vi "日志信息出发送队列 (子VI).vi"() -> (0 "错误输出":errorcluster)   [LabVIEW 2016, in "数据传输系统-03.lvlib"]
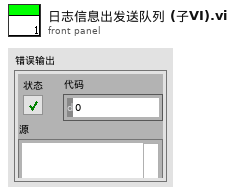
[diagram p1: front panel]
types:
  T1 = enum16{"空白测试", "跨度核查", "标样核查", "加标回收", "平行样", "集成干预"}
  T2 = cluster{"氨氮零点核查索引起始时间":string, "总磷零点核查索引起始时间":string, "总氮零点核查索引起始时间":string, "CODMn零点核查索引起始时间":string, "CODCr零点核查索引起始时间":string, "亚硝酸盐零点核查索引起始时间":string, "硫化物零点核查索引起始时间":string, "ORP零点核查索引起始时间":string, "氟化物零点核查索引起始时间":string}
  T3 = cluster{"数组[0]":string, "数组[1]":string, "数组[2]":string, "数组[3]":string, "数组[4]":string, "数组[5]":string, "数组[6]":string, "数组[7]":string, "数组[8]":string}
  T4 = cluster{"PH":string[][], "CODCr":string[][], "氨氮":string[][], "CODMn":string[][], "总氮":string[][], "总磷":string[][], "电导率":string[][], "水温":string[][], "DO":string[][], "浊度":string[][], "叶绿素":string[][], "藻密度":string[][], "铜":string[][], "盐度":string[][], "水位":string[][], "流速":string[][], "瞬时流量":string[][], "累积流量":string[][], "亚硝酸盐":string[][], "硫化物":string[][], "ORP":string[][], "铅":string[][], "镉":string[][], "锌":string[][], "镍":string[][], "锰":string[][], "汞":string[][], "气温":string[][], "气压":string[][], "风速":string[][], "风向":string[][], "盐度 2":string[][], "磷酸盐":string[][], "硝氮":string[][], "氟化物":string[][]}
  T5 = cluster{"氨氮跨度核查索引起始时间":string, "总磷跨度核查索引起始时间":string, "总氮跨度核查索引起始时间":string, "CODMn跨度核查索引起始时间":string, "CODCr跨度核查索引起始时间":string, "亚硝酸盐跨度核查索引起始时间":string, "硫化物跨度核查索引起始时间":string, "ORP跨度核查索引起始时间":string, "氟化物跨度核查索引起始时间":string}
  T6 = cluster{"氨氮标样核查索引起始时间":string, "总磷标样核查索引起始时间":string, "总氮标样核查索引起始时间":string, "CODMn标样核查索引起始时间":string, "CODCr标样核查索引起始时间":string, "DO标样核查索引起始时间":string, "PH标样核查索引起始时间":string, "比电导率标样核查索引起始时间":string, "水温标样核查索引起始时间":string, "浊度标样核查索引起始时间":string, "叶绿素a标样核查索引起始时间":string, "藻密度标样核查索引起始时间":string, "亚硝酸盐标样核查索引起始时间":string, "硫化物标样核查索引起始时间":string, "ORP标样核查索引起始时间":string, "氟化物标样核查索引起始时间":string}
  T7 = cluster{"数组[0]":string, "数组[1]":string, "数组[2]":string, "数组[3]":string, "数组[4]":string, "数组[5]":string, "数组[6]":string, "数组[7]":string, "数组[8]":string, "数组[9]":string, "数组[10]":string, "数组[11]":string, "数组[12]":string, "数组[13]":string, "数组[14]":string, "数组[15]":string}
  T8 = cluster{"氨氮加标回收索引起始时间":string, "总磷加标回收索引起始时间":string, "总氮加标回收索引起始时间":string, "CODMn加标回收索引起始时间":string, "CODCr加标回收索引起始时间":string, "氟化物加标回收索引起始时间":string}
  T9 = cluster{"[0]":string, "[1]":string, "[2]":string, "[3]":string, "[4]":string, "[5]":string}
  T10 = cluster{"氨氮平行样索引起始时间":string, "总磷平行样索引起始时间":string, "总氮平行样索引起始时间":string, "CODMn平行样索引起始时间":string, "CODCr平行样索引起始时间":string, "氟化物平行样索引起始时间":string}
  T11 = cluster{"氨氮集成干预索引起始时间":string, "总磷集成干预索引起始时间":string, "总氮集成干预索引起始时间":string, "CODMn集成干预索引起始时间":string, "CODCr集成干预索引起始时间":string, "DO集成干预索引起始时间":string, "PH集成干预索引起始时间":string, "比电导率集成干预索引起始时间":string, "水温集成干预索引起始时间":string, "浊度集成干预索引起始时间":string, "叶绿素a集成干预索引起始时间":string, "藻密度集成干预索引起始时间":string, "亚硝酸盐集成干预索引起始时间":string, "硫化物集成干预索引起始时间":string, "ORP集成干预索引起始时间":string, "氟化物集成干预索引起始时间":string}
  T12 = cluster{"[0]":string, "[1]":string, "[2]":string, "[3]":string, "[4]":string, "[5]":string, "[6]":string, "[7]":string, "[8]":string, "[9]":string, "[10]":string, "[11]":string, "[12]":string, "[13]":string, "[14]":string, "[15]":string}
  T13 = cluster{"氨氮仪器日志索引起始时间":string, "总磷仪器日志索引起始时间":string, "总氮仪器日志索引起始时间":string, "CODMn仪器日志索引起始时间":string, "CODCr仪器日志索引起始时间":string, "系统仪器日志索引起始时间":string, "氟化物仪器日志索引起始时间":string}
  T14 = cluster{"[0]":string, "[1]":string, "[2]":string, "[3]":string, "[4]":string, "[5]":string, "[6]":string}
  T15 = cluster{"氨氮报警信息索引起始时间":string, "总磷报警信息索引起始时间":string, "总氮报警信息索引起始时间":string, "CODMn报警信息索引起始时间":string, "CODCr报警信息索引起始时间":string, "DO报警信息索引起始时间":string, "PH报警信息索引起始时间":string, "比电导率报警信息索引起始时间":string, "水温报警信息索引起始时间":string, "浊度报警信息索引起始时间":string, "叶绿素报警信息索引起始时间":string, "系统报警信息索引起始时间":string, "氟化物报警信息索引起始时间":string}
  T16 = cluster{"[0]":string, "[1]":string, "[2]":string, "[3]":string, "[4]":string, "[5]":string, "[6]":string, "[7]":string, "[8]":string, "[9]":string, "[10]":string, "[11]":string, "[12]":string}
  T17 = cluster{"氨氮仪器参数索引起始时间":string, "总磷仪器参数索引起始时间":string, "总氮仪器参数索引起始时间":string, "CODMn仪器参数索引起始时间":string, "CODCr仪器参数索引起始时间":string, "DO仪器参数索引起始时间":string, "PH仪器参数索引起始时间":string, "比电导率仪器参数索引起始时间":string, "水温仪器参数索引起始时间":string, "浊度仪器参数索引起始时间":string, "叶绿素a仪器参数索引起始时间":string, "藻密度仪器参数索引起始时间":string, "ORP仪器参数索引起始时间":string, "氟化物仪器参数索引起始时间":string}
  T18 = cluster{"[0]":string, "[1]":string, "[2]":string, "[3]":string, "[4]":string, "[5]":string, "[6]":string, "[7]":string, "[8]":string, "[9]":string, "[10]":string, "[11]":string, "[12]":string, "[13]":string}
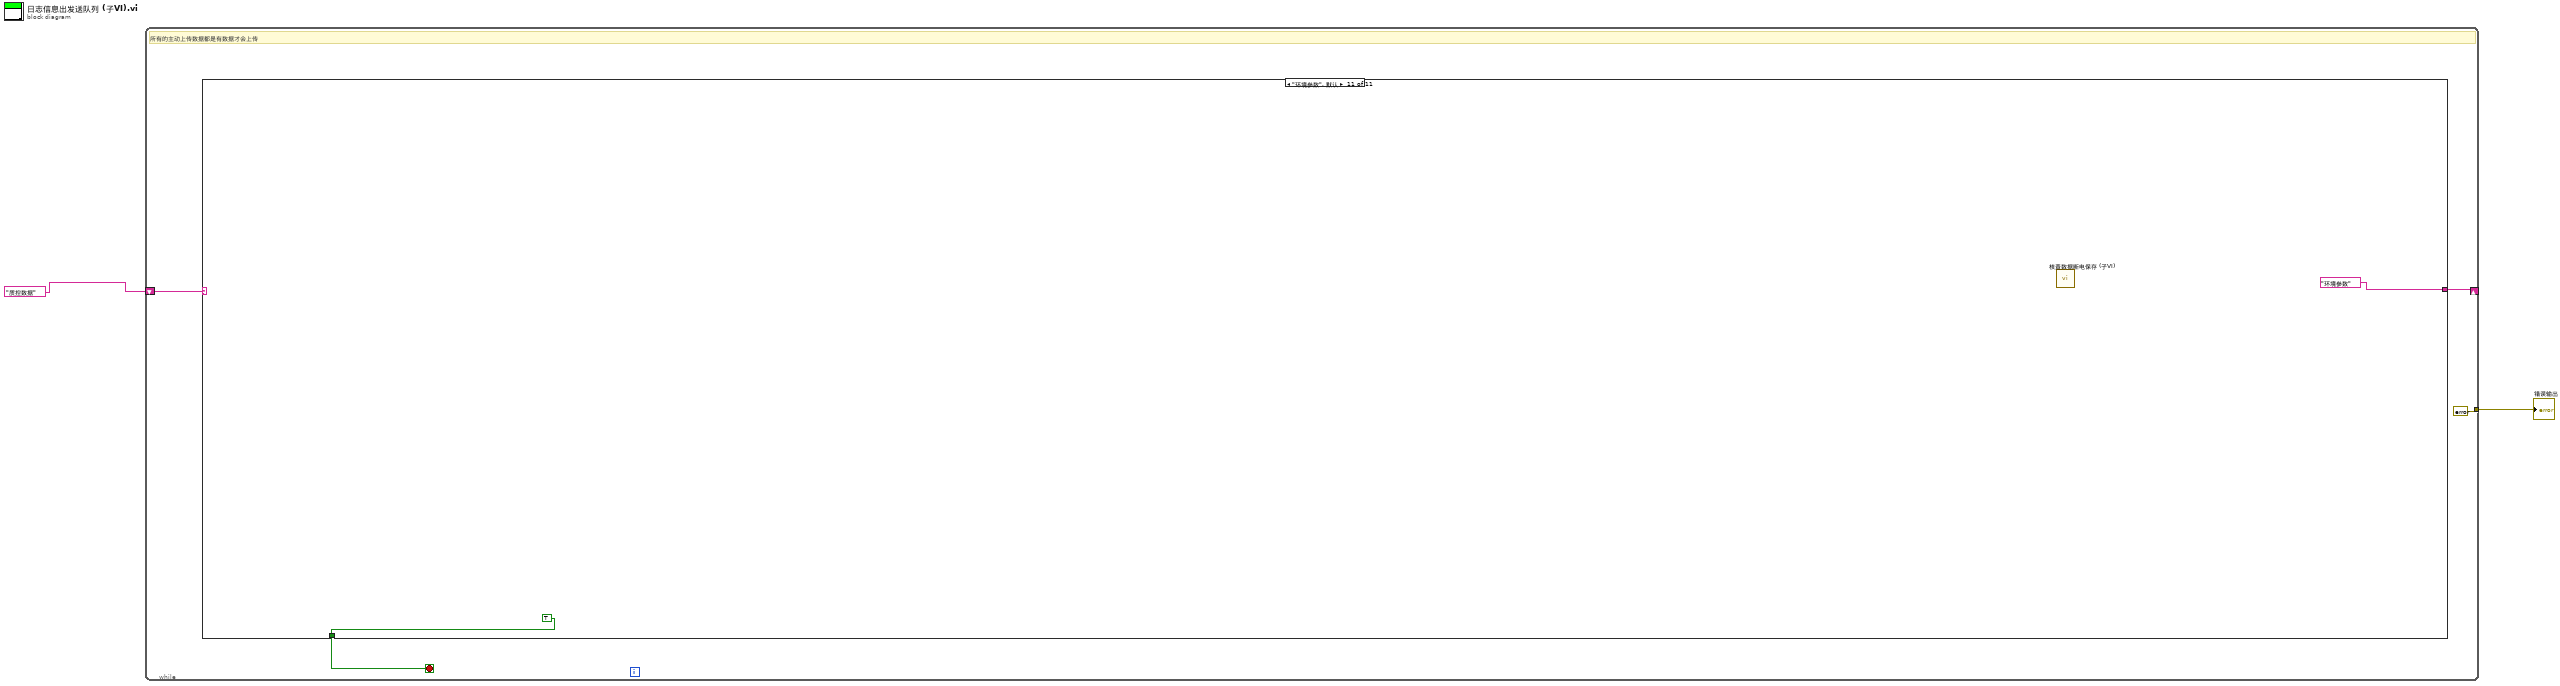
[diagram p0: block diagram]
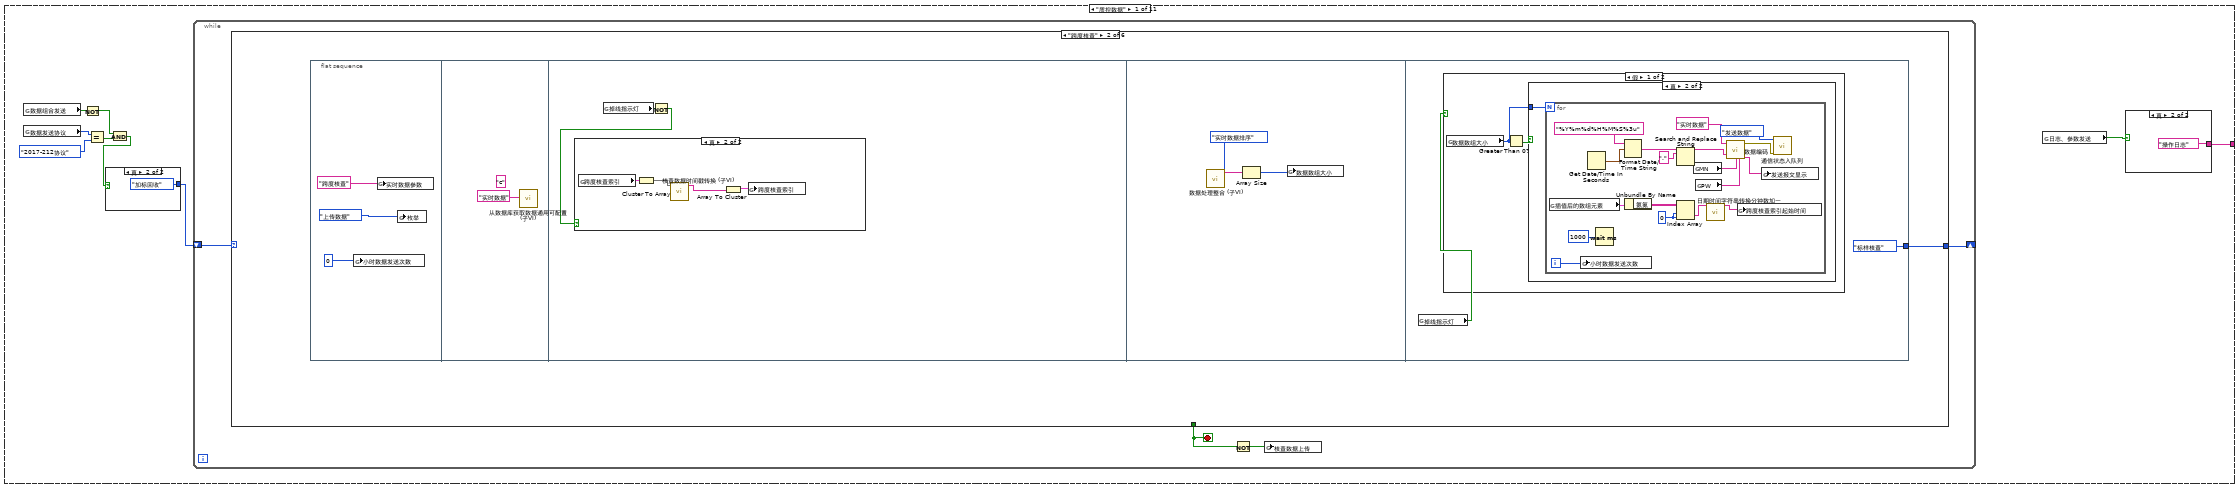
[diagram p2: hidden frame]
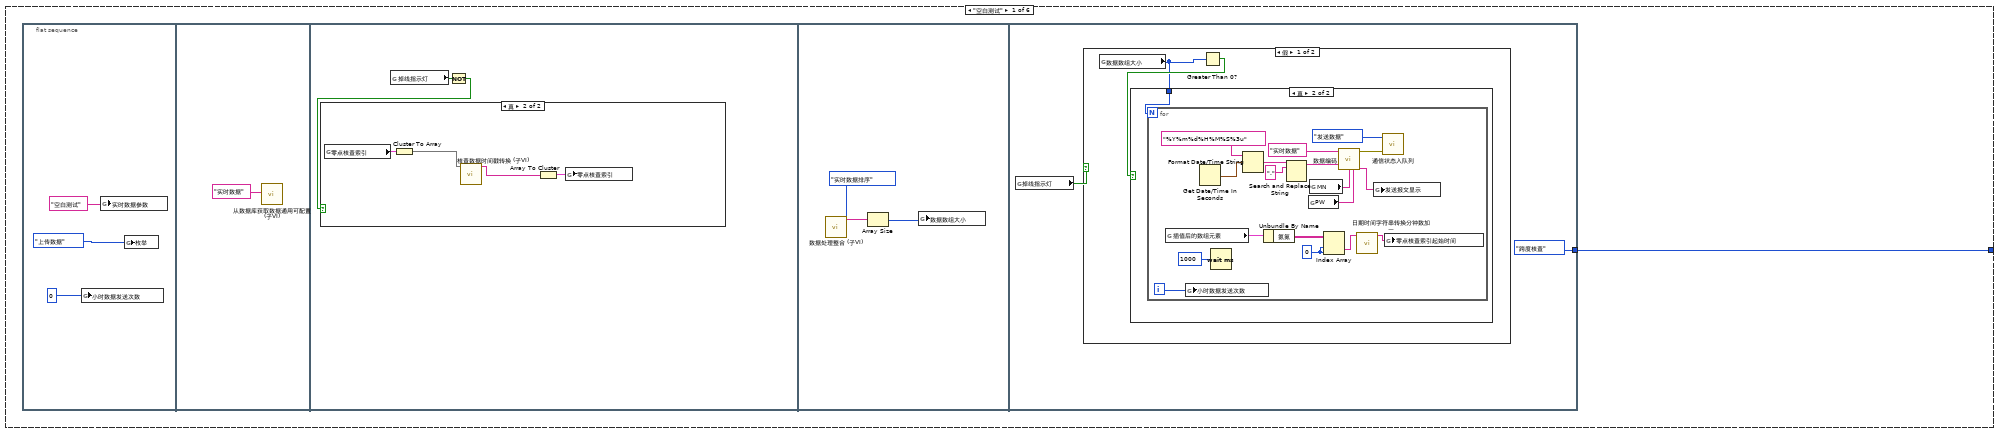
[diagram p3: hidden frame]
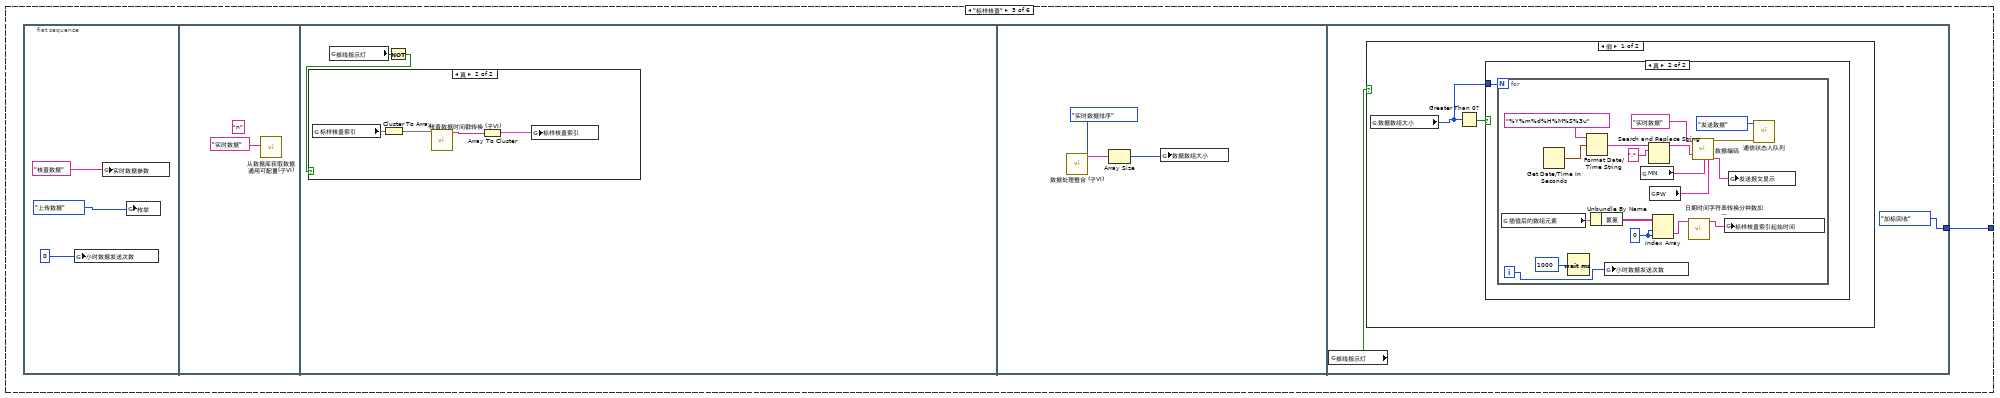
[diagram p10: hidden frame]
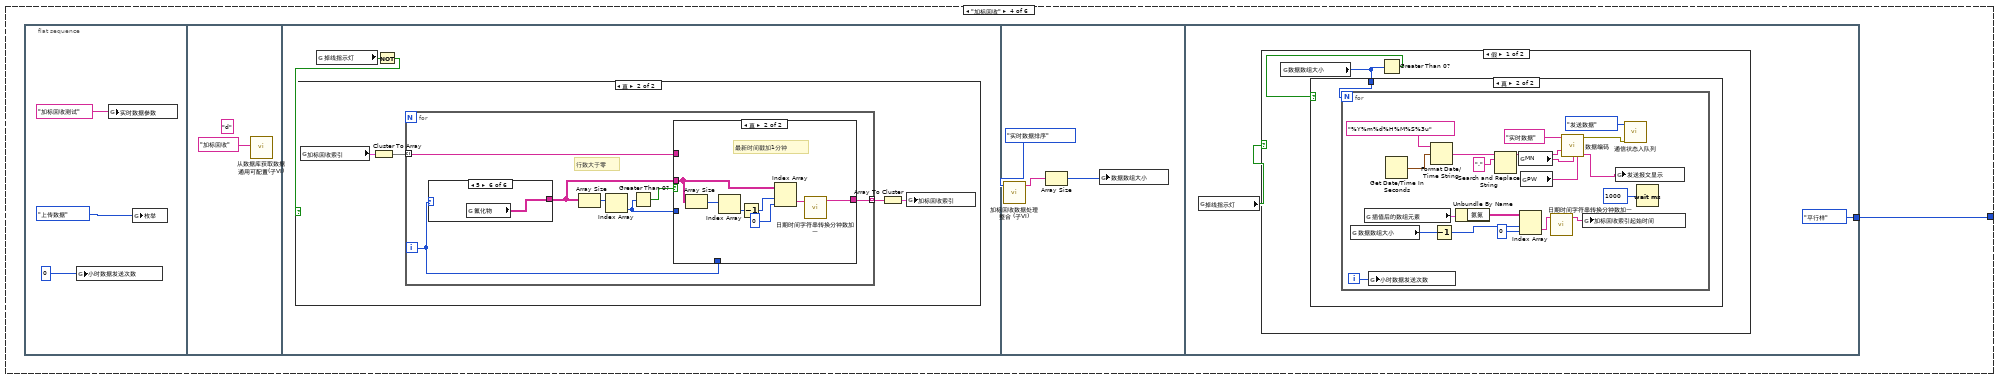
[diagram p14: hidden frame]
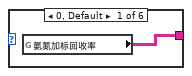
[diagram p16: hidden frame]
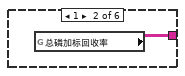
[diagram p17: hidden frame]
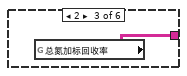
[diagram p18: hidden frame]
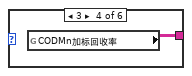
[diagram p19: hidden frame]
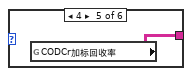
[diagram p20: hidden frame]
diagram:
  n1 = while "While循环" {
    shift-right: [w5] -> _
    shift-left: "质控数据" ("组合框") -> [w6]
    tunnel: [errorcluster {"status"=FALSE, "code"=0, "source"=""} ("错误输出")] -> w2
    stop <- w3 stop-if-true
    # "所有的主动上传数据都是有数据才会上传"
    n2 = case shown="\"环境参数\", 默认" w6 {
      tunnel: [w15 w312 "系统状态" ("组合框") w414 "测量周期" ("组合框") "超标留样" ("组合框") "报警信息" ("组合框") w508 w574 "环境参数" ("组合框") "环境参数" ("组合框")] -> w5
      tunnel: [_ _ _ _ _ _ _ _ _ _ TRUE] -> w3
      frame "质控数据" {
        n3 = global read "断电保存全局.vi" "数据组合发送"() -> (w10:bool)
        n4 = global read "断电保存全局.vi" "数据发送协议"() -> (w13:enum16{"2005-212协议", "2017-212协议"})
        n5 = Not(x=w10) -> (.not. x?=w9:bool)
        n6 = Equal?(x=w13, y=enum16{"2005-212协议", "2017-212协议"}."2017-212协议" ("数据发送协议")) -> (x = y?=w11:bool)
        n7 = And(x=w9, y=w11) -> (x .and. y?=w8:bool)
        n8 = case shown="真" w8 {
          tunnel: [T1."空白测试" T1."加标回收"] -> w7
          frame False {
          }
          frame True {
          }
        }
        n9 = while {
          shift-right: [w18] -> _
          shift-left: w7 -> [w19]
          stop <- w16 stop-if-true
          n10 = case shown="\"跨度核查\"" w19 {
            tunnel: [_ _ _ _ _ TRUE] -> w16
            tunnel: [w20 w57 w94 w131 w191 w244] -> w18
            frame "空白测试" {
              n11 = flat-sequence {
                tunnel: [T1."跨度核查"] -> w20
                frame #0 {
                  n12 = global write "全局 小时数据发送次数.vi" "小时数据发送次数"(0 ("小时数据发送次数")) -> ()
                  n13 = global write "全局 实时数据参数.vi" "实时数据参数"("空白测试") -> ()
                  n14 = global write "全局1.vi" "枚举"(enum16{"返回请求应答", "上传数据", "返回执行结果"}."上传数据" ("枚举")) -> ()
                }
                frame #1 {
                  n15 = call "从数据库获取数据通用可配置(子VI).vi"("table输入"="实时数据" ("新元素/子数组")) -> ()  [unwired: 9 in, 2 out]
                }
                frame #2 {
                  n16 = global read "全局 数据发送重叠.vi" "掉线指示灯"() -> (w26:bool)
                  n17 = Not(x=w26) -> (.not. x?=w25:bool)
                  n18 = case shown="真" w25 {
                    frame False {
                    }
                    frame True {
                      n19 = global read "全局 时间2.vi" "零点核查索引"() -> (w30:T2)
                      n20 = Cluster To Array(cluster=w30) -> (array=w28:string[])
                      n21 = call "核查数据时间戳转换 (子VI).vi"("核查索引"=w28) -> ("数组"=w27:string[])  [unwired: 10 in]
                      n22 = Array To Cluster(array=w27) -> (cluster=w29:T3)
                      n23 = global write "全局 时间2.vi" "零点核查索引"(w29) -> ()
                    }
                  }
                }
                frame #3 {
                  n24 = call "数据处理整合 (子VI).vi"("枚举"=enum16{"实时数据排序", "小时数据排序"}."实时数据排序") -> ("已排序的数组"=w33:string[])  [unwired: 10 in]
                  n25 = Array Size(array=w33) -> (size(s)=w32:i32)
                  n26 = global write "全局 数据数组大小.vi" "数据数组大小"(w32) -> ()
                }
                frame #4 {
                  n27 = global read "全局 数据发送重叠.vi" "掉线指示灯"() -> (w35:bool)
                  n28 = case shown="假" w35 {
                    frame False {
                      n29 = global read "全局 数据数组大小.vi" "数据数组大小"() -> (w36:i32)
                      n30 = Greater Than 0?(x=w36) -> (x > 0?=w37:bool)
                      n31 = case shown="真" w37 {
                        tunnel: w36 -> [_ w38]
                        frame False {
                        }
                        frame True {
                          n32 = for {
                            N: w38 -> [_]
                            i -> [w39]
                            w51 = 0 ("禁用的索引 (列)")
                            n33 = global read "插值后的新数组.vi" "插值后的数组元素"() -> (w55:T4)
                            n34 = global write "全局 小时数据发送次数.vi" "小时数据发送次数"(w39) -> ()
                            n35 = Get Date/Time In Seconds() -> (seconds since 1Jan1904=w43:timestamp)
                            n36 = Wait (ms)(milliseconds to wait=u32 1000 ("等待时间（毫秒）")) -> ()  [unwired: 1 out]
                            n37 = Format Date/Time String(time format string (%c)="%Y%m%d%H%M%S%3u" ("时间格式字符串(%c)"), seconds (now)=w43) -> (date/time string=w42:string)  [unwired: 1 in]
                            n38 = Unbundle By Name(w55) -> ("氨氮"=w54:string[][])
                            n39 = Search and Replace String(input string=w42, search string="." ("搜索字符串")) -> (result string=w40:string)  [unwired: 6 in, 3 out]
                            n40 = global read "断电保存全局.vi" "PW"() -> (w47:string)
                            n41 = global read "断电保存全局.vi" "MN"() -> (w48:string)
                            n42 = Index Array(array=w54, index (row)=w51, index (col)=w51) -> (element=w53:string)
                            n43 = call "数据编码.vi"("table输入"="实时数据" ("新元素/子数组"), "QN"=w40, "MN"=w48, "PW"=w47) -> ("错误常量"=w46:errorcluster, "通讯包字符串"=w50:string)  [unwired: 10 in]
                            n44 = call "日期时间字符串转换分钟数加一.vi"("data[0]"=w53) -> ("日期/时间字符串"=w52:string)  [unwired: 10 in]
                            n45 = global write "全局1.vi" "发送报文显示"(w50) -> ()
                            n46 = call "通信状态入队列.vi"("错误输入（无错误）"=w46, "枚举"=enum16{"打开连接", "发送数据", "读取数据", "数据处理", "关闭连接"}."发送数据") -> ()  [unwired: 9 in, 1 out]
                            n47 = global write "全局 时间2.vi" "零点核查索引起始时间"(w52) -> ()
                          }
                        }
                      }
                    }
                    frame True {
                    }
                  }
                }
              }
            }
            frame "跨度核查" {
              n48 = flat-sequence {
                tunnel: [T1."标样核查"] -> w57
                frame #0 {
                  n49 = global write "全局 小时数据发送次数.vi" "小时数据发送次数"(0 ("小时数据发送次数")) -> ()
                  n50 = global write "全局 实时数据参数.vi" "实时数据参数"("跨度核查") -> ()
                  n51 = global write "全局1.vi" "枚举"(enum16{"返回请求应答", "上传数据", "返回执行结果"}."上传数据" ("枚举")) -> ()
                }
                frame #1 {
                  (unwired) "c" ("列队名（唯一）")
                  n52 = call "从数据库获取数据通用可配置(子VI).vi"("table输入"="实时数据" ("新元素/子数组")) -> ()  [unwired: 9 in, 2 out]
                }
                frame #2 {
                  n53 = global read "全局 数据发送重叠.vi" "掉线指示灯"() -> (w63:bool)
                  n54 = Not(x=w63) -> (.not. x?=w62:bool)
                  n55 = case shown="真" w62 {
                    frame False {
                    }
                    frame True {
                      n56 = global read "全局 时间2.vi" "跨度核查索引"() -> (w67:T5)
                      n57 = Cluster To Array(cluster=w67) -> (array=w65:string[])
                      n58 = call "核查数据时间戳转换 (子VI).vi"("核查索引"=w65) -> ("数组"=w64:string[])  [unwired: 10 in]
                      n59 = Array To Cluster(array=w64) -> (cluster=w66:T3)
                      n60 = global write "全局 时间2.vi" "跨度核查索引"(w66) -> ()
                    }
                  }
                }
                frame #3 {
                  n61 = call "数据处理整合 (子VI).vi"("枚举"=enum16{"实时数据排序", "小时数据排序"}."实时数据排序") -> ("已排序的数组"=w70:string[])  [unwired: 10 in]
                  n62 = Array Size(array=w70) -> (size(s)=w69:i32)
                  n63 = global write "全局 数据数组大小.vi" "数据数组大小"(w69) -> ()
                }
                frame #4 {
                  n64 = global read "全局 数据发送重叠.vi" "掉线指示灯"() -> (w72:bool)
                  n65 = case shown="假" w72 {
                    frame False {
                      n66 = global read "全局 数据数组大小.vi" "数据数组大小"() -> (w73:i32)
                      n67 = Greater Than 0?(x=w73) -> (x > 0?=w74:bool)
                      n68 = case shown="真" w74 {
                        tunnel: w73 -> [_ w75]
                        frame False {
                        }
                        frame True {
                          n69 = for {
                            N: w75 -> [_]
                            i -> [w76]
                            w88 = 0 ("禁用的索引 (列)")
                            n70 = global read "插值后的新数组.vi" "插值后的数组元素"() -> (w92:T4)
                            n71 = global write "全局 小时数据发送次数.vi" "小时数据发送次数"(w76) -> ()
                            n72 = Get Date/Time In Seconds() -> (seconds since 1Jan1904=w80:timestamp)
                            n73 = Wait (ms)(milliseconds to wait=u32 1000 ("等待时间（毫秒）")) -> ()  [unwired: 1 out]
                            n74 = Format Date/Time String(time format string (%c)="%Y%m%d%H%M%S%3u" ("时间格式字符串(%c)"), seconds (now)=w80) -> (date/time string=w79:string)  [unwired: 1 in]
                            n75 = Unbundle By Name(w92) -> ("氨氮"=w91:string[][])
                            n76 = Index Array(array=w91, index (row)=w88, index (col)=w88) -> (element=w90:string)
                            n77 = Search and Replace String(input string=w79, search string="." ("搜索字符串")) -> (result string=w77:string)  [unwired: 6 in, 3 out]
                            n78 = global read "断电保存全局.vi" "MN"() -> (w86:string)
                            n79 = global read "断电保存全局.vi" "PW"() -> (w85:string)
                            n80 = call "日期时间字符串转换分钟数加一.vi"("data[0]"=w90) -> ("日期/时间字符串"=w89:string)  [unwired: 10 in]
                            n81 = call "数据编码.vi"("table输入"="实时数据" ("新元素/子数组"), "QN"=w77, "MN"=w86, "PW"=w85) -> ("错误常量"=w83:errorcluster, "通讯包字符串"=w84:string)  [unwired: 10 in]
                            n82 = global write "全局 时间2.vi" "跨度核查索引起始时间"(w89) -> ()
                            n83 = global write "全局1.vi" "发送报文显示"(w84) -> ()
                            n84 = call "通信状态入队列.vi"("错误输入（无错误）"=w83, "枚举"=enum16{"打开连接", "发送数据", "读取数据", "数据处理", "关闭连接"}."发送数据") -> ()  [unwired: 9 in, 1 out]
                          }
                        }
                      }
                    }
                    frame True {
                    }
                  }
                }
              }
            }
            frame "标样核查" {
              n85 = flat-sequence {
                tunnel: [T1."加标回收"] -> w94
                frame #0 {
                  n86 = global write "全局 小时数据发送次数.vi" "小时数据发送次数"(0 ("小时数据发送次数")) -> ()
                  n87 = global write "全局 实时数据参数.vi" "实时数据参数"("核查数据") -> ()
                  n88 = global write "全局1.vi" "枚举"(enum16{"返回请求应答", "上传数据", "返回执行结果"}."上传数据" ("枚举")) -> ()
                }
                frame #1 {
                  (unwired) "n" ("列队名（唯一）")
                  n89 = call "从数据库获取数据通用可配置(子VI).vi"("table输入"="实时数据" ("新元素/子数组")) -> ()  [unwired: 9 in, 2 out]
                }
                frame #2 {
                  n90 = global read "全局 数据发送重叠.vi" "掉线指示灯"() -> (w100:bool)
                  n91 = Not(x=w100) -> (.not. x?=w99:bool)
                  n92 = case shown="真" w99 {
                    frame False {
                    }
                    frame True {
                      n93 = global read "全局 时间2.vi" "标样核查索引"() -> (w104:T6)
                      n94 = Cluster To Array(cluster=w104) -> (array=w102:string[])
                      n95 = call "核查数据时间戳转换 (子VI).vi"("核查索引"=w102) -> ("数组"=w101:string[])  [unwired: 10 in]
                      n96 = Array To Cluster(array=w101) -> (cluster=w103:T7)
                      n97 = global write "全局 时间2.vi" "标样核查索引"(w103) -> ()
                    }
                  }
                }
                frame #3 {
                  n98 = call "数据处理整合 (子VI).vi"("枚举"=enum16{"实时数据排序", "小时数据排序"}."实时数据排序") -> ("已排序的数组"=w107:string[])  [unwired: 10 in]
                  n99 = Array Size(array=w107) -> (size(s)=w106:i32)
                  n100 = global write "全局 数据数组大小.vi" "数据数组大小"(w106) -> ()
                }
                frame #4 {
                  n101 = global read "全局 数据发送重叠.vi" "掉线指示灯"() -> (w109:bool)
                  n102 = case shown="假" w109 {
                    frame False {
                      n103 = global read "全局 数据数组大小.vi" "数据数组大小"() -> (w110:i32)
                      n104 = Greater Than 0?(x=w110) -> (x > 0?=w111:bool)
                      n105 = case shown="真" w111 {
                        tunnel: w110 -> [_ w112]
                        frame False {
                        }
                        frame True {
                          n106 = for {
                            N: w112 -> [_]
                            i -> [w113]
                            w125 = 0 ("禁用的索引 (列)")
                            n107 = global read "插值后的新数组.vi" "插值后的数组元素"() -> (w129:T4)
                            n108 = Get Date/Time In Seconds() -> (seconds since 1Jan1904=w117:timestamp)
                            n109 = Wait (ms)(milliseconds to wait=u32 1000 ("等待时间（毫秒）")) -> ()  [unwired: 1 out]
                            n110 = Format Date/Time String(time format string (%c)="%Y%m%d%H%M%S%3u" ("时间格式字符串(%c)"), seconds (now)=w117) -> (date/time string=w116:string)  [unwired: 1 in]
                            n111 = Unbundle By Name(w129) -> ("氨氮"=w128:string[][])
                            n112 = global write "全局 小时数据发送次数.vi" "小时数据发送次数"(w113) -> ()
                            n113 = global read "断电保存全局.vi" "MN"() -> (w122:string)
                            n114 = Search and Replace String(input string=w116, search string="." ("搜索字符串")) -> (result string=w114:string)  [unwired: 6 in, 3 out]
                            n115 = global read "断电保存全局.vi" "PW"() -> (w121:string)
                            n116 = Index Array(array=w128, index (row)=w125, index (col)=w125) -> (element=w127:string)
                            n117 = call "日期时间字符串转换分钟数加一.vi"("data[0]"=w127) -> ("日期/时间字符串"=w126:string)  [unwired: 10 in]
                            n118 = call "数据编码.vi"("table输入"="实时数据" ("新元素/子数组"), "QN"=w114, "MN"=w122, "PW"=w121) -> ("错误常量"=w120:errorcluster, "通讯包字符串"=w124:string)  [unwired: 10 in]
                            n119 = global write "全局 时间2.vi" "标样核查索引起始时间"(w126) -> ()
                            n120 = global write "全局1.vi" "发送报文显示"(w124) -> ()
                            n121 = call "通信状态入队列.vi"("错误输入（无错误）"=w120, "枚举"=enum16{"打开连接", "发送数据", "读取数据", "数据处理", "关闭连接"}."发送数据") -> ()  [unwired: 9 in, 1 out]
                          }
                        }
                      }
                    }
                    frame True {
                    }
                  }
                }
              }
            }
            frame "加标回收" {
              n122 = flat-sequence {
                tunnel: [T1."平行样"] -> w131
                frame #0 {
                  n123 = global write "全局 小时数据发送次数.vi" "小时数据发送次数"(0 ("小时数据发送次数")) -> ()
                  n124 = global write "全局 实时数据参数.vi" "实时数据参数"("加标回收测试") -> ()
                  n125 = global write "全局1.vi" "枚举"(enum16{"返回请求应答", "上传数据", "返回执行结果"}."上传数据" ("枚举")) -> ()
                }
                frame #1 {
                  (unwired) "d" ("列队名（唯一）")
                  n126 = call "从数据库获取数据通用可配置(子VI).vi"("table输入"="加标回收" ("新元素/子数组")) -> ()  [unwired: 9 in, 2 out]
                }
                frame #2 {
                  n127 = global read "全局 数据发送重叠.vi" "掉线指示灯"() -> (w137:bool)
                  n128 = Not(x=w137) -> (.not. x?=w136:bool)
                  n129 = case shown="真" w136 {
                    frame False {
                    }
                    frame True {
                      n130 = global read "全局 时间2.vi" "加标回收索引"() -> (w141:T8)
                      n131 = Cluster To Array(cluster=w141) -> (array=w140:string[])
                      n132 = for {
                        tunnel: [w143] -> w138 mode=indexing
                        tunnel: w140 -> [w142] mode=indexing
                        i -> [w144]
                        # "行数大于零"
                        n133 = case shown="5" w144 {
                          tunnel: [w149 w150 w151 w152 w153 w154] -> w145
                          frame 0, Default {
                            n134 = global read "全局 所有参数.vi" "氨氮加标回收率"() -> (w149:string[][])
                          }
                          frame 1 {
                            n135 = global read "全局 所有参数.vi" "总磷加标回收率"() -> (w150:string[][])
                          }
                          frame 2 {
                            n136 = global read "全局 所有参数.vi" "总氮加标回收率"() -> (w151:string[][])
                          }
                          frame 3 {
                            n137 = global read "全局 所有参数.vi" "CODMn加标回收率"() -> (w152:string[][])
                          }
                          frame 4 {
                            n138 = global read "全局 所有参数.vi" "CODCr加标回收率"() -> (w153:string[][])
                          }
                          frame 5 {
                            n139 = global read "全局 所有参数.vi" "氟化物"() -> (w154:string[][])
                          }
                        }
                        n140 = Array Size(array=w145) -> (size(s)=w147:i32[])
                        n141 = Index Array(array=w147) -> (element=w146:i32)  [unwired: 1 in]
                        n142 = Greater Than 0?(x=w146) -> (x > 0?=w148:bool)
                        n143 = case shown="真" w148 {
                          tunnel: w144 -> [_ _]
                          tunnel: w146 -> [_ _]
                          tunnel: w145 -> [_ w159]
                          tunnel: [w155 w156] -> w143
                          tunnel: w142 -> [w155 _]
                          frame False {
                          }
                          frame True {
                            # "最新时间戳加1分钟"
                            n144 = Array Size(array=w159) -> (size(s)=w161:i32[])
                            n145 = Index Array(array=w161) -> (element=w160:i32)  [unwired: 1 in]
                            n146 = Decrement(x=w160) -> (x-1=w158:i32)
                            n147 = Index Array(array=w159, index (row)=w158, index (col)=0 ("禁用的索引 (列)")) -> (element=w162:string)
                            n148 = call "日期时间字符串转换分钟数加一.vi"("data[0]"=w162) -> ("日期/时间字符串"=w156:string)  [unwired: 10 in]
                          }
                        }
                      }
                      n149 = Array To Cluster(array=w138) -> (cluster=w139:T9)
                      n150 = global write "全局 时间2.vi" "加标回收索引"(w139) -> ()
                    }
                  }
                }
                frame #3 {
                  n151 = call "加标回收数据处理整合 (子VI).vi"("枚举"=enum16{"实时数据排序", "小时数据排序"}."实时数据排序") -> ("已排序的数组"=w164:string[])  [unwired: 10 in]
                  n152 = Array Size(array=w164) -> (size(s)=w165:i32)
                  n153 = global write "全局 数据数组大小.vi" "数据数组大小"(w165) -> ()
                }
                frame #4 {
                  n154 = global read "全局 数据发送重叠.vi" "掉线指示灯"() -> (w167:bool)
                  n155 = case shown="假" w167 {
                    frame False {
                      n156 = global read "全局 数据数组大小.vi" "数据数组大小"() -> (w168:i32)
                      n157 = Greater Than 0?(x=w168) -> (x > 0?=w169:bool)
                      n158 = case shown="真" w169 {
                        tunnel: w168 -> [_ w170]
                        frame False {
                        }
                        frame True {
                          n159 = for {
                            N: w170 -> [_]
                            i -> [w171]
                            n160 = global read "全局 数据数组大小.vi" "数据数组大小"() -> (w186:i32)
                            n161 = global read "插值后的新数组.vi" "插值后的数组元素"() -> (w189:T4)
                            n162 = global write "全局 小时数据发送次数.vi" "小时数据发送次数"(w171) -> ()
                            n163 = Get Date/Time In Seconds() -> (seconds since 1Jan1904=w175:timestamp)
                            n164 = Format Date/Time String(time format string (%c)="%Y%m%d%H%M%S%3u" ("时间格式字符串(%c)"), seconds (now)=w175) -> (date/time string=w174:string)  [unwired: 1 in]
                            n165 = Decrement(x=w186) -> (x-1=w185:i32)
                            n166 = Unbundle By Name(w189) -> ("氨氮"=w188:string[][])
                            n167 = Search and Replace String(input string=w174, search string="." ("搜索字符串")) -> (result string=w172:string)  [unwired: 6 in, 3 out]
                            n168 = global read "断电保存全局.vi" "MN"() -> (w180:string)
                            n169 = Index Array(array=w188, index (row)=w185, index (col)=0 ("禁用的索引 (列)")) -> (element=w184:string)
                            n170 = global read "断电保存全局.vi" "PW"() -> (w179:string)
                            n171 = call "日期时间字符串转换分钟数加一.vi"("data[0]"=w184) -> ("日期/时间字符串"=w183:string)  [unwired: 10 in]
                            n172 = call "数据编码.vi"("table输入"="实时数据" ("新元素/子数组"), "QN"=w172, "MN"=w180, "PW"=w179) -> ("错误常量"=w178:errorcluster, "通讯包字符串"=w182:string)  [unwired: 10 in]
                            n173 = global write "全局 时间2.vi" "加标回收索引起始时间"(w183) -> ()
                            n174 = global write "全局1.vi" "发送报文显示"(w182) -> ()
                            n175 = call "通信状态入队列.vi"("错误输入（无错误）"=w178, "枚举"=enum16{"打开连接", "发送数据", "读取数据", "数据处理", "关闭连接"}."发送数据") -> ()  [unwired: 9 in, 1 out]
                            n176 = Wait (ms)(milliseconds to wait=u32 1000 ("等待时间（毫秒）")) -> ()  [unwired: 1 out]
                          }
                        }
                      }
                    }
                    frame True {
                    }
                  }
                }
              }
            }
            frame "平行样" {
              n177 = flat-sequence {
                tunnel: [T1."集成干预"] -> w191
                frame #0 {
                  n178 = global write "全局 小时数据发送次数.vi" "小时数据发送次数"(0 ("小时数据发送次数")) -> ()
                  n179 = global write "全局 实时数据参数.vi" "实时数据参数"("平行样测试") -> ()
                  n180 = global write "全局1.vi" "枚举"(enum16{"返回请求应答", "上传数据", "返回执行结果"}."上传数据" ("枚举")) -> ()
                }
                frame #1 {
                  (unwired) "e" ("列队名（唯一）")
                  n181 = call "从数据库获取数据通用可配置(子VI).vi"("table输入"="平行样测试" ("新元素/子数组")) -> ()  [unwired: 9 in, 2 out]
                }
                frame #2 {
                  n182 = global read "全局 数据发送重叠.vi" "掉线指示灯"() -> (w197:bool)
                  n183 = Not(x=w197) -> (.not. x?=w196:bool)
                  n184 = case shown="真" w196 {
                    frame False {
                    }
                    frame True {
                      n185 = global read "全局 时间2.vi" "平行样索引"() -> (w201:T10)
                      n186 = Cluster To Array(cluster=w201) -> (array=w200:string[])
                      n187 = for {
                        tunnel: [w203] -> w198 mode=indexing
                        tunnel: w200 -> [w202] mode=indexing
                        i -> [w204]
                        # "行数大于零"
                        n188 = case shown="5" w204 {
                          tunnel: [w209 w210 w211 w212 w213 w214] -> w205
                          frame 0, Default {
                            n189 = global read "全局 所有参数.vi" "氨氮"() -> (w209:string[][])
                          }
                          frame 1 {
                            n190 = global read "全局 所有参数.vi" "总磷"() -> (w210:string[][])
                          }
                          frame 2 {
                            n191 = global read "全局 所有参数.vi" "总氮"() -> (w211:string[][])
                          }
                          frame 3 {
                            n192 = global read "全局 所有参数.vi" "CODMn"() -> (w212:string[][])
                          }
                          frame 4 {
                            n193 = global read "全局 所有参数.vi" "CODCr"() -> (w213:string[][])
                          }
                          frame 5 {
                            n194 = global read "全局 所有参数.vi" "氟化物"() -> (w214:string[][])
                          }
                        }
                        n195 = Array Size(array=w205) -> (size(s)=w207:i32[])
                        n196 = Index Array(array=w207) -> (element=w206:i32)  [unwired: 1 in]
                        n197 = Greater Than 0?(x=w206) -> (x > 0?=w208:bool)
                        n198 = case shown="真" w208 {
                          tunnel: w204 -> [_ _]
                          tunnel: w206 -> [_ _]
                          tunnel: w205 -> [_ w219]
                          tunnel: [w215 w216] -> w203
                          tunnel: w202 -> [w215 _]
                          frame False {
                          }
                          frame True {
                            # "最新时间戳加1分钟"
                            n199 = Array Size(array=w219) -> (size(s)=w221:i32[])
                            n200 = Index Array(array=w221) -> (element=w220:i32)  [unwired: 1 in]
                            n201 = Decrement(x=w220) -> (x-1=w218:i32)
                            n202 = Index Array(array=w219, index (row)=w218, index (col)=0 ("禁用的索引 (列)")) -> (element=w222:string)
                            n203 = call "日期时间字符串转换分钟数加一.vi"("data[0]"=w222) -> ("日期/时间字符串"=w216:string)  [unwired: 10 in]
                          }
                        }
                      }
                      n204 = Array To Cluster(array=w198) -> (cluster=w199:T9)
                      n205 = global write "全局 时间2.vi" "平行样索引"(w199) -> ()
                    }
                  }
                }
                frame #3 {
                  n206 = call "数据处理整合 (子VI).vi"("枚举"=enum16{"实时数据排序", "小时数据排序"}."实时数据排序") -> ("已排序的数组"=w225:string[])  [unwired: 10 in]
                  n207 = Array Size(array=w225) -> (size(s)=w224:i32)
                  n208 = global write "全局 数据数组大小.vi" "数据数组大小"(w224) -> ()
                }
                frame #4 {
                  n209 = global read "全局 数据发送重叠.vi" "掉线指示灯"() -> (w226:bool)
                  n210 = case shown="假" w226 {
                    frame False {
                      n211 = global read "全局 数据数组大小.vi" "数据数组大小"() -> (w228:i32)
                      n212 = Greater Than 0?(x=w228) -> (x > 0?=w229:bool)
                      n213 = case shown="真" w229 {
                        tunnel: w228 -> [_ w230]
                        frame False {
                        }
                        frame True {
                          n214 = for {
                            N: w230 -> [_]
                            i -> [w231]
                            n215 = global write "全局 小时数据发送次数.vi" "小时数据发送次数"(w231) -> ()
                            n216 = Get Date/Time In Seconds() -> (seconds since 1Jan1904=w235:timestamp)
                            n217 = Format Date/Time String(time format string (%c)="%Y%m%d%H%M%S%3u" ("时间格式字符串(%c)"), seconds (now)=w235) -> (date/time string=w234:string)  [unwired: 1 in]
                            n218 = Search and Replace String(input string=w234, search string="." ("搜索字符串")) -> (result string=w232:string)  [unwired: 6 in, 3 out]
                            n219 = global read "断电保存全局.vi" "MN"() -> (w240:string)
                            n220 = global read "断电保存全局.vi" "PW"() -> (w239:string)
                            n221 = call "数据编码.vi"("table输入"="实时数据" ("新元素/子数组"), "QN"=w232, "MN"=w240, "PW"=w239) -> ("错误常量"=w238:errorcluster, "通讯包字符串"=w242:string)  [unwired: 10 in]
                            n222 = global write "全局1.vi" "发送报文显示"(w242) -> ()
                            n223 = call "通信状态入队列.vi"("错误输入（无错误）"=w238, "枚举"=enum16{"打开连接", "发送数据", "读取数据", "数据处理", "关闭连接"}."发送数据") -> ()  [unwired: 9 in, 1 out]
                            n224 = Wait (ms)(milliseconds to wait=u32 1000 ("等待时间（毫秒）")) -> ()  [unwired: 1 out]
                          }
                        }
                      }
                    }
                    frame True {
                    }
                  }
                }
              }
            }
            frame "集成干预" {
              n225 = flat-sequence {
                tunnel: [T1."集成干预"] -> w244
                frame #0 {
                  n226 = global write "全局 小时数据发送次数.vi" "小时数据发送次数"(0 ("小时数据发送次数")) -> ()
                  n227 = global write "全局 实时数据参数.vi" "实时数据参数"("集成干预测试") -> ()
                  n228 = global write "全局1.vi" "枚举"(enum16{"返回请求应答", "上传数据", "返回执行结果"}."上传数据" ("枚举")) -> ()
                }
                frame #1 {
                  (unwired) "f" ("列队名（唯一）")
                  n229 = call "从数据库获取数据通用可配置(子VI).vi"("table输入"="集成干预测试" ("新元素/子数组")) -> ()  [unwired: 9 in, 2 out]
                }
                frame #2 {
                  n230 = global read "全局 数据发送重叠.vi" "掉线指示灯"() -> (w251:bool)
                  n231 = Not(x=w251) -> (.not. x?=w250:bool)
                  n232 = case shown="真" w250 {
                    frame False {
                    }
                    frame True {
                      n233 = global read "全局 时间2.vi" "集成干预索引"() -> (w255:T11)
                      n234 = Cluster To Array(cluster=w255) -> (array=w254:string[])
                      n235 = for {
                        tunnel: [w257] -> w252 mode=indexing
                        tunnel: w254 -> [w256] mode=indexing
                        i -> [w258]
                        # "行数大于零"
                        n236 = case shown="15" w258 {
                          tunnel: [w263 w264 w265 w266 w267 w268 w269 w270 w271 w272 w273 w274 w275 w276 w277 w278] -> w259
                          frame 0, Default {
                            n237 = global read "全局 所有参数.vi" "氨氮"() -> (w263:string[][])
                          }
                          frame 1 {
                            n238 = global read "全局 所有参数.vi" "总磷"() -> (w264:string[][])
                          }
                          frame 2 {
                            n239 = global read "全局 所有参数.vi" "总氮"() -> (w265:string[][])
                          }
                          frame 3 {
                            n240 = global read "全局 所有参数.vi" "CODMn"() -> (w266:string[][])
                          }
                          frame 4 {
                            n241 = global read "全局 所有参数.vi" "CODCr"() -> (w267:string[][])
                          }
                          frame 5 {
                            n242 = global read "全局 所有参数.vi" "DO"() -> (w268:string[][])
                          }
                          frame 6 {
                            n243 = global read "全局 所有参数.vi" "PH"() -> (w269:string[][])
                          }
                          frame 7 {
                            n244 = global read "全局 所有参数.vi" "电导率"() -> (w270:string[][])
                          }
                          frame 8 {
                            n245 = global read "全局 所有参数.vi" "水温"() -> (w271:string[][])
                          }
                          frame 9 {
                            n246 = global read "全局 所有参数.vi" "浊度"() -> (w272:string[][])
                          }
                          frame 10 {
                            n247 = global read "全局 所有参数.vi" "叶绿素"() -> (w273:string[][])
                          }
                          frame 11 {
                            n248 = global read "全局 所有参数.vi" "藻密度"() -> (w274:string[][])
                          }
                          frame 12 {
                            n249 = global read "全局 所有参数.vi" "亚硝酸盐"() -> (w275:string[][])
                          }
                          frame 13 {
                            n250 = global read "全局 所有参数.vi" "硫化物"() -> (w276:string[][])
                          }
                          frame 14 {
                            n251 = global read "全局 所有参数.vi" "ORP"() -> (w277:string[][])
                          }
                          frame 15 {
                            n252 = global read "全局 所有参数.vi" "氟化物"() -> (w278:string[][])
                          }
                        }
                        n253 = Array Size(array=w259) -> (size(s)=w261:i32[])
                        n254 = Index Array(array=w261) -> (element=w260:i32)  [unwired: 1 in]
                        n255 = Greater Than 0?(x=w260) -> (x > 0?=w262:bool)
                        n256 = case shown="真" w262 {
                          tunnel: w258 -> [_ _]
                          tunnel: w260 -> [_ _]
                          tunnel: w259 -> [_ w281]
                          tunnel: [w279 w280] -> w257
                          tunnel: w256 -> [w279 _]
                          frame False {
                          }
                          frame True {
                            # "最新时间戳加1分钟"
                            n257 = Array Size(array=w281) -> (size(s)=w285:i32[])
                            n258 = Index Array(array=w285) -> (element=w284:i32)  [unwired: 1 in]
                            n259 = Decrement(x=w284) -> (x-1=w283:i32)
                            n260 = Index Array(array=w281, index (row)=w283, index (col)=0 ("禁用的索引 (列)")) -> (element=w286:string)
                            n261 = call "日期时间字符串转换分钟数加一.vi"("data[0]"=w286) -> ("日期/时间字符串"=w280:string)  [unwired: 10 in]
                          }
                        }
                      }
                      n262 = Array To Cluster(array=w252) -> (cluster=w253:T12)
                      n263 = global write "全局 时间2.vi" "集成干预索引"(w253) -> ()
                    }
                  }
                }
                frame #3 {
                  n264 = call "数据处理整合 (子VI).vi"("枚举"=enum16{"实时数据排序", "小时数据排序"}."实时数据排序") -> ("已排序的数组"=w289:string[])  [unwired: 10 in]
                  n265 = Array Size(array=w289) -> (size(s)=w288:i32)
                  n266 = global write "全局 数据数组大小.vi" "数据数组大小"(w288) -> ()
                }
                frame #4 {
                  n267 = global read "全局 数据发送重叠.vi" "掉线指示灯"() -> (w291:bool)
                  n268 = case shown="假" w291 {
                    frame False {
                      n269 = global read "全局 数据数组大小.vi" "数据数组大小"() -> (w292:i32)
                      n270 = Greater Than 0?(x=w292) -> (x > 0?=w293:bool)
                      n271 = case shown="真" w293 {
                        tunnel: w292 -> [_ w294]
                        frame False {
                        }
                        frame True {
                          n272 = for {
                            N: w294 -> [_]
                            i -> [w295]
                            n273 = Get Date/Time In Seconds() -> (seconds since 1Jan1904=w299:timestamp)
                            n274 = Format Date/Time String(time format string (%c)="%Y%m%d%H%M%S%3u" ("时间格式字符串(%c)"), seconds (now)=w299) -> (date/time string=w298:string)  [unwired: 1 in]
                            n275 = global write "全局 小时数据发送次数.vi" "小时数据发送次数"(w295) -> ()
                            n276 = global read "断电保存全局.vi" "MN"() -> (w303:string)
                            n277 = global read "断电保存全局.vi" "PW"() -> (w302:string)
                            n278 = Search and Replace String(input string=w298, search string="." ("搜索字符串")) -> (result string=w296:string)  [unwired: 6 in, 3 out]
                            n279 = call "数据编码.vi"("table输入"="实时数据" ("新元素/子数组"), "QN"=w296, "MN"=w303, "PW"=w302) -> ("错误常量"=w304:errorcluster, "通讯包字符串"=w306:string)  [unwired: 10 in]
                            n280 = global write "全局1.vi" "发送报文显示"(w306) -> ()
                            n281 = call "通信状态入队列.vi"("错误输入（无错误）"=w304, "枚举"=enum16{"打开连接", "发送数据", "读取数据", "数据处理", "关闭连接"}."发送数据") -> ()  [unwired: 9 in, 1 out]
                            n282 = Wait (ms)(milliseconds to wait=u32 1000 ("等待时间（毫秒）")) -> ()  [unwired: 1 out]
                          }
                        }
                      }
                    }
                    frame True {
                    }
                  }
                }
              }
            }
          }
          n283 = Not(x=w16) -> (.not. x?=w17:bool)
          n284 = global write "全局1.vi" "核查数据上传"(w17) -> ()
        }
        n285 = global read "断电保存全局.vi" "日志、参数发送"() -> (w14:bool)
        n286 = case shown="真" w14 {
          tunnel: ["环境参数" ("组合框") "操作日志" ("组合框")] -> w15
          frame False {
          }
          frame True {
          }
        }
      }
      frame "操作日志" {
        # "间隔时间上传"
        # "直接1分钟查询 一次,有数据就按数据上传,没数据就不上传,在数据发送那边有做处理"
        n287 = flat-sequence {
          frame #0 {
            # "时间"
            n288 = global write "全局 小时数据发送次数.vi" "小时数据发送次数"(0 ("小时数据发送次数")) -> ()
            n289 = call "日志信息主动发送(子VI).vi"() -> ()  [unwired: 12 in]
            n290 = global write "全局1.vi" "枚举"(enum16{"返回请求应答", "上传数据", "返回执行结果"}."上传数据" ("枚举")) -> ()
          }
          frame #1 {
            n291 = call "获取操作日志 (子VI).vi"("table输入"="操作日志") -> ()  [unwired: 11 in]
          }
          frame #2 {
            n292 = call "数据处理整合 (子VI).vi"("枚举"=enum16{"实时数据排序", "小时数据排序"}."实时数据排序") -> ("已排序的数组"=w321:string[])  [unwired: 10 in]
            n293 = Array Size(array=w321) -> (size(s)=w320:i32)
            n294 = global write "全局 数据数组大小.vi" "数据数组大小"(w320) -> ()
          }
          frame #3 {
            n295 = global read "全局 数据发送重叠.vi" "掉线指示灯"() -> (w323:bool)
            n296 = Not(x=w323) -> (.not. x?=w322:bool)
            n297 = case shown="真" w322 {
              frame False {
              }
              frame True {
                n298 = global read "全局 时间2.vi" "仪器日志索引"() -> (w327:T13)
                n299 = Cluster To Array(cluster=w327) -> (array=w326:string[])
                n300 = for {
                  tunnel: w326 -> [w328] mode=indexing
                  tunnel: [w329] -> w324 mode=indexing
                  i -> [w331]
                  # "行数大于零"
                  n301 = case shown="6" w331 {
                    tunnel: [w335 w336 w337 w338 w339 w340 w341] -> w330
                    frame 0, Default {
                      n302 = global read "全局 所有参数.vi" "氨氮"() -> (w335:string[][])
                    }
                    frame 1 {
                      n303 = global read "全局 所有参数.vi" "总磷"() -> (w336:string[][])
                    }
                    frame 2 {
                      n304 = global read "全局 所有参数.vi" "总氮"() -> (w337:string[][])
                    }
                    frame 3 {
                      n305 = global read "全局 所有参数.vi" "CODMn"() -> (w338:string[][])
                    }
                    frame 4 {
                      n306 = global read "全局 所有参数.vi" "CODCr"() -> (w339:string[][])
                    }
                    frame 5 {
                      n307 = global read "全局 所有参数.vi" "DO"() -> (w340:string[][])
                    }
                    frame 6 {
                      n308 = global read "全局 所有参数.vi" "氟化物"() -> (w341:string[][])
                    }
                  }
                  n309 = Array Size(array=w330) -> (size(s)=w333:i32[])
                  n310 = Index Array(array=w333) -> (element=w332:i32)  [unwired: 1 in]
                  n311 = Greater Than 0?(x=w332) -> (x > 0?=w334:bool)
                  n312 = case shown="真" w334 {
                    tunnel: w332 -> [_ _]
                    tunnel: w330 -> [_ w347]
                    tunnel: [w342 w343] -> w329
                    tunnel: w328 -> [w342 _]
                    frame False {
                    }
                    frame True {
                      # "最新时间戳加1分钟"
                      n313 = Array Size(array=w347) -> (size(s)=w349:i32[])
                      n314 = Index Array(array=w349) -> (element=w348:i32)  [unwired: 1 in]
                      n315 = Decrement(x=w348) -> (x-1=w346:i32)
                      n316 = Index Array(array=w347, index (row)=w346, index (col)=0 ("禁用的索引 (列)")) -> (element=w344:string)
                      n317 = call "日期时间字符串转换秒数加一.vi"("data[0]"=w344) -> ("日期/时间字符串"=w343:string)  [unwired: 10 in]
                    }
                  }
                }
                n318 = Array To Cluster(array=w324) -> (cluster=w325:T14)
                n319 = global write "全局 时间2.vi" "仪器日志索引"(w325) -> ()
              }
            }
          }
          frame #4 {
            # "判定是否存表"
            n320 = global read "全局 数据发送重叠.vi" "掉线指示灯"() -> (w350:bool)
            n321 = case shown="假" w350 {
              frame False {
                n322 = global read "全局 数据数组大小.vi" "数据数组大小"() -> (w351:i32)
                n323 = Greater Than 0?(x=w351) -> (x > 0?=w352:bool)
                n324 = case shown="真" w352 {
                  frame False {
                  }
                  frame True {
                    n325 = while {
                      stop <- w354 stop-if-true
                      n326 = Get Date/Time In Seconds() -> (seconds since 1Jan1904=w366:timestamp)
                      n327 = Format Date/Time String(time format string (%c)="%Y%m%d%H%M%S%3u" ("时间格式字符串(%c)"), seconds (now)=w366) -> (date/time string=w365:string)  [unwired: 1 in]
                      n328 = Search and Replace String(input string=w365, search string="." ("搜索字符串")) -> (result string=w363:string)  [unwired: 6 in, 3 out]
                      n329 = global read "断电保存全局.vi" "MN"() -> (w360:string)
                      n330 = global read "断电保存全局.vi" "PW"() -> (w359:string)
                      n331 = call "数据编码.vi"("table输入"="操作日志" ("新元素/子数组"), "QN"=w363, "MN"=w360, "PW"=w359) -> ("错误常量"=w358:errorcluster, "通讯包字符串"=w362:string)  [unwired: 10 in]
                      n332 = global read "全局 小时数据发送次数.vi" "小时数据发送次数"() -> (w355:i32)
                      n333 = global read "全局 数据数组大小.vi" "数据数组大小"() -> (w356:i32)
                      n334 = call "通信状态入队列.vi"("错误输入（无错误）"=w358, "枚举"=enum16{"打开连接", "发送数据", "读取数据", "数据处理", "关闭连接"}."发送数据") -> ()  [unwired: 9 in, 1 out]
                      n335 = global write "全局1.vi" "发送报文显示"(w362) -> ()
                      n336 = Decrement(x=w356) -> (x-1=w357:i32)
                      n337 = Greater Or Equal?(x=w355, y=w357) -> (x >= y?=w354:bool)
                      n338 = Wait (ms)(milliseconds to wait=u32 1000 ("等待时间（毫秒）")) -> ()  [unwired: 1 out]
                    }
                  }
                }
              }
              frame True {
              }
            }
          }
        }
        n339 = global read "断电保存全局.vi" "应用环境"() -> (w313:enum16{"STD", "GB212"})
        n340 = case shown="\"STD\", 默认" w313 {
          tunnel: ["3092日志信息" ("组合框") "系统状态" ("组合框")] -> w312
          frame "STD", Default {
          }
          frame "GB212" {
          }
        }
      }
      frame "3092日志信息" {
        # "间隔时间上传"
        # "直接1分钟查询 一次,有数据就按数据上传,没数据就不上传,在数据发送那边有做处理"
        n341 = flat-sequence {
          tunnel: [w373] -> w369
          tunnel: w369 -> [w377]
          frame #0 {
            n342 = global write "全局 小时数据发送次数.vi" "小时数据发送次数"(0 ("小时数据发送次数")) -> ()
            n343 = global write "全局1.vi" "枚举"(enum16{"返回请求应答", "上传数据", "返回执行结果"}."上传数据" ("枚举")) -> ()
          }
          frame #1 {
            n344 = call "数据表比对.vi"("table输入"="3092日志信息") -> ("待发送数据"=w373:string[][])  [unwired: 7 in, 3 out]
            n345 = global write "全局 所有参数.vi" "CODMn"(w373) -> ()
          }
          frame #2 {
            n346 = Array Size(array=w377) -> (size(s)=w376:i32[])
            n347 = Index Array(array=w376) -> (element=w375:i32)  [unwired: 1 in]
            n348 = global write "全局 数据数组大小.vi" "数据数组大小"(w375) -> ()
          }
          frame #3 {
            n349 = global read "全局 数据发送重叠.vi" "掉线指示灯"() -> (w379:bool)
            n350 = Not(x=w379) -> (.not. x?=w378:bool)
            n351 = case shown="真" w378 {
              frame False {
              }
              frame True {
                # "行数大于零"
                n352 = global read "全局 时间2.vi" "3092日志索引起始时间"() -> (w381:string)
                n353 = global read "全局 所有参数.vi" "CODMn"() -> (w382:string[][])
                n354 = Array Size(array=w382) -> (size(s)=w384:i32[])
                n355 = Index Array(array=w384) -> (element=w383:i32)  [unwired: 1 in]
                n356 = Greater Than 0?(x=w383) -> (x > 0?=w385:bool)
                n357 = case shown="真" w385 {
                  tunnel: w383 -> [_ _]
                  tunnel: w382 -> [_ w391]
                  tunnel: [w386 w387] -> w380
                  tunnel: w381 -> [w386 _]
                  frame False {
                  }
                  frame True {
                    # "最新时间戳加1分钟"
                    n358 = Array Size(array=w391) -> (size(s)=w393:i32[])
                    n359 = Index Array(array=w393) -> (element=w392:i32)  [unwired: 1 in]
                    n360 = Decrement(x=w392) -> (x-1=w390:i32)
                    n361 = Index Array(array=w391, index (row)=w390, index (col)=0 ("禁用的索引 (列)")) -> (element=w388:string)
                    n362 = call "日期时间字符串转换秒数加一.vi"("data[0]"=w388) -> ("日期/时间字符串"=w387:string)  [unwired: 10 in]
                  }
                }
                n363 = global write "全局 时间2.vi" "3092日志索引起始时间"(w380) -> ()
              }
            }
          }
          frame #4 {
            # "判定是否存表"
            n364 = global read "全局 数据发送重叠.vi" "掉线指示灯"() -> (w394:bool)
            n365 = case shown="假" w394 {
              frame False {
                n366 = global read "全局 数据数组大小.vi" "数据数组大小"() -> (w395:i32)
                n367 = Greater Than 0?(x=w395) -> (x > 0?=w396:bool)
                n368 = case shown="真" w396 {
                  frame False {
                  }
                  frame True {
                    n369 = while {
                      stop <- w398 stop-if-true
                      n370 = global read "全局 数据数组大小.vi" "数据数组大小"() -> (w400:i32)
                      n371 = Wait (ms)(milliseconds to wait=u32 1000 ("等待时间（毫秒）")) -> ()  [unwired: 1 out]
                      n372 = global read "全局 小时数据发送次数.vi" "小时数据发送次数"() -> (w399:i32)
                      n373 = Decrement(x=w400) -> (x-1=w401:i32)
                      n374 = Greater Or Equal?(x=w399, y=w401) -> (x >= y?=w398:bool)
                      n375 = Get Date/Time In Seconds() -> (seconds since 1Jan1904=w410:timestamp)
                      n376 = Format Date/Time String(time format string (%c)="%Y%m%d%H%M%S%3u" ("时间格式字符串(%c)"), seconds (now)=w410) -> (date/time string=w409:string)  [unwired: 1 in]
                      n377 = Search and Replace String(input string=w409, search string="." ("搜索字符串")) -> (result string=w407:string)  [unwired: 6 in, 3 out]
                      n378 = global read "断电保存全局.vi" "MN"() -> (w404:string)
                      n379 = global read "断电保存全局.vi" "PW"() -> (w403:string)
                      n380 = call "数据编码.vi"("table输入"="3092日志信息" ("新元素/子数组"), "QN"=w407, "MN"=w404, "PW"=w403) -> ("错误常量"=w402:errorcluster, "通讯包字符串"=w406:string)  [unwired: 10 in]
                      n381 = call "通信状态入队列.vi"("错误输入（无错误）"=w402, "枚举"=enum16{"打开连接", "发送数据", "读取数据", "数据处理", "关闭连接"}."发送数据") -> ()  [unwired: 9 in, 1 out]
                      n382 = global write "全局1.vi" "发送报文显示"(w406) -> ()
                    }
                  }
                }
              }
              frame True {
              }
            }
          }
        }
      }
      frame "系统状态" {
        # "直接1分钟查询 一次,有变化就按上传,没变化就不上传"
        n383 = flat-sequence {
          frame #0 {
            # "时间"
            n384 = global write "全局 小时数据发送次数.vi" "小时数据发送次数"(0 ("小时数据发送次数")) -> ()
            n385 = global write "全局 数据数组大小.vi" "数据数组大小"(1 ("数据数组大小")) -> ()
            n386 = global write "全局1.vi" "枚举"(enum16{"返回请求应答", "上传数据", "返回执行结果"}."上传数据" ("枚举")) -> ()
          }
          frame #1 {
            # "判定是否存表"
            n387 = global read "全局 数据发送重叠.vi" "掉线指示灯"() -> (w420:bool)
            n388 = case shown="假" w420 {
              frame False {
                n389 = global read "全局1.vi" "系统状态"() -> (w421:bool)
                n390 = case shown="真" w421 {
                  frame False {
                  }
                  frame True {
                    n391 = for {
                      N: 6 -> [_]
                      n392 = flat-sequence {
                        frame #0 {
                          n393 = Get Date/Time In Seconds() -> (seconds since 1Jan1904=w433:timestamp)
                          n394 = Format Date/Time String(time format string (%c)="%Y%m%d%H%M%S%3u" ("时间格式字符串(%c)"), seconds (now)=w433) -> (date/time string=w432:string)  [unwired: 1 in]
                          n395 = Search and Replace String(input string=w432, search string="." ("搜索字符串")) -> (result string=w430:string)  [unwired: 6 in, 3 out]
                          n396 = global read "断电保存全局.vi" "MN"() -> (w427:string)
                          n397 = global read "断电保存全局.vi" "PW"() -> (w426:string)
                          n398 = call "数据编码.vi"("table输入"="系统状态" ("新元素/子数组"), "QN"=w430, "MN"=w427, "PW"=w426) -> ("错误常量"=w425:errorcluster, "通讯包字符串"=w429:string)  [unwired: 10 in]
                          n399 = global write "全局1.vi" "发送报文显示"(w429) -> ()
                          n400 = call "通信状态入队列.vi"("错误输入（无错误）"=w425, "枚举"=enum16{"打开连接", "发送数据", "读取数据", "数据处理", "关闭连接"}."发送数据") -> ()  [unwired: 9 in, 1 out]
                        }
                        frame #1 {
                          n401 = global read "全局 小时数据发送次数.vi" "小时数据发送次数"() -> (w437:i32)
                          n402 = Increment(x=w437) -> (x+1=w436:i32)
                          n403 = global write "全局 小时数据发送次数.vi" "小时数据发送次数"(w436) -> ()
                        }
                      }
                      n404 = Wait (ms)(milliseconds to wait=u32 1000 ("等待时间（毫秒）")) -> ()  [unwired: 1 out]
                    }
                    n405 = global write "全局1.vi" "系统状态"(FALSE ("系统状态")) -> ()
                  }
                }
              }
              frame True {
              }
            }
          }
        }
        n406 = global read "断电保存全局.vi" "应用环境"() -> (w413:enum16{"STD", "GB212"})
        n407 = case shown="\"GB212\"" w413 {
          tunnel: ["运行模式" ("组合框") "超标留样" ("组合框")] -> w414
          frame "STD", Default {
          }
          frame "GB212" {
          }
        }
      }
      frame "运行模式" {
        # "直接1分钟查询 一次,有变化就按上传,没变化就不上传"
        n408 = flat-sequence {
          frame #0 {
            # "时间"
            n409 = global write "全局 小时数据发送次数.vi" "小时数据发送次数"(0 ("小时数据发送次数")) -> ()
            n410 = global write "全局 数据数组大小.vi" "数据数组大小"(1 ("数据数组大小")) -> ()
            n411 = global write "全局1.vi" "枚举"(enum16{"返回请求应答", "上传数据", "返回执行结果"}."上传数据" ("枚举")) -> ()
          }
          frame #1 {
            # "判定是否存表"
            n412 = global read "全局 数据发送重叠.vi" "掉线指示灯"() -> (w442:bool)
            n413 = case shown="假" w442 {
              frame False {
                n414 = global read "全局1.vi" "运行模式"() -> (w443:bool)
                n415 = case shown="真" w443 {
                  frame False {
                  }
                  frame True {
                    n416 = global read "全局 小时数据发送次数.vi" "小时数据发送次数"() -> (w451:i32)
                    n417 = global write "全局1.vi" "运行模式"(FALSE ("系统状态")) -> ()
                    n418 = Get Date/Time In Seconds() -> (seconds since 1Jan1904=w455:timestamp)
                    n419 = Increment(x=w451) -> (x+1=w450:i32)
                    n420 = Format Date/Time String(time format string (%c)="%Y%m%d%H%M%S%3u" ("时间格式字符串(%c)"), seconds (now)=w455) -> (date/time string=w454:string)  [unwired: 1 in]
                    n421 = global write "全局 小时数据发送次数.vi" "小时数据发送次数"(w450) -> ()
                    n422 = Search and Replace String(input string=w454, search string="." ("搜索字符串")) -> (result string=w452:string)  [unwired: 6 in, 3 out]
                    n423 = global read "断电保存全局.vi" "MN"() -> (w447:string)
                    n424 = global read "断电保存全局.vi" "PW"() -> (w446:string)
                    n425 = call "数据编码.vi"("table输入"="运行模式" ("新元素/子数组"), "QN"=w452, "MN"=w447, "PW"=w446) -> ("错误常量"=w445:errorcluster, "通讯包字符串"=w449:string)  [unwired: 10 in]
                    n426 = call "通信状态入队列.vi"("错误输入（无错误）"=w445, "枚举"=enum16{"打开连接", "发送数据", "读取数据", "数据处理", "关闭连接"}."发送数据") -> ()  [unwired: 9 in, 1 out]
                    n427 = global write "全局1.vi" "发送报文显示"(w449) -> ()
                  }
                }
              }
              frame True {
              }
            }
          }
        }
      }
      frame "测量周期" {
        # "直接1分钟查询 一次,有变化就按上传,没变化就不上传"
        n428 = flat-sequence {
          frame #0 {
            # "时间"
            n429 = global write "全局 小时数据发送次数.vi" "小时数据发送次数"(0 ("小时数据发送次数")) -> ()
            n430 = global write "全局 数据数组大小.vi" "数据数组大小"(1 ("数据数组大小")) -> ()
            n431 = global write "全局1.vi" "枚举"(enum16{"返回请求应答", "上传数据", "返回执行结果"}."上传数据" ("枚举")) -> ()
          }
          frame #1 {
            # "判定是否存表"
            n432 = global read "全局 数据发送重叠.vi" "掉线指示灯"() -> (w462:bool)
            n433 = case shown="假" w462 {
              frame False {
                n434 = global read "全局1.vi" "测量周期"() -> (w463:bool)
                n435 = case shown="真" w463 {
                  frame False {
                  }
                  frame True {
                    n436 = flat-sequence {
                      frame #0 {
                        n437 = Get Date/Time In Seconds() -> (seconds since 1Jan1904=w473:timestamp)
                        n438 = Format Date/Time String(time format string (%c)="%Y%m%d%H%M%S%3u" ("时间格式字符串(%c)"), seconds (now)=w473) -> (date/time string=w472:string)  [unwired: 1 in]
                        n439 = global read "断电保存全局.vi" "MN"() -> (w467:string)
                        n440 = global read "断电保存全局.vi" "PW"() -> (w466:string)
                        n441 = Search and Replace String(input string=w472, search string="." ("搜索字符串")) -> (result string=w470:string)  [unwired: 6 in, 3 out]
                        n442 = call "数据编码.vi"("table输入"="测量周期" ("新元素/子数组"), "QN"=w470, "MN"=w467, "PW"=w466) -> ("错误常量"=w465:errorcluster, "通讯包字符串"=w469:string)  [unwired: 10 in]
                        n443 = call "通信状态入队列.vi"("错误输入（无错误）"=w465, "枚举"=enum16{"打开连接", "发送数据", "读取数据", "数据处理", "关闭连接"}."发送数据") -> ()  [unwired: 9 in, 1 out]
                        n444 = global write "全局1.vi" "发送报文显示"(w469) -> ()
                      }
                      frame #1 {
                        n445 = Wait (ms)(milliseconds to wait=u32 1000 ("等待时间（毫秒）")) -> ()  [unwired: 1 out]
                      }
                      frame #2 {
                        n446 = Get Date/Time In Seconds() -> (seconds since 1Jan1904=w479:timestamp)
                        n447 = Format Date/Time String(time format string (%c)="%Y%m%d%H%M%S%3u" ("时间格式字符串(%c)"), seconds (now)=w479) -> (date/time string=w480:string)  [unwired: 1 in]
                        n448 = global read "断电保存全局.vi" "MN"() -> (w485:string)
                        n449 = global read "断电保存全局.vi" "PW"() -> (w486:string)
                        n450 = Search and Replace String(input string=w480, search string="." ("搜索字符串")) -> (result string=w482:string)  [unwired: 6 in, 3 out]
                        n451 = call "数据编码.vi"("table输入"="各参数测量周期" ("新元素/子数组"), "QN"=w482, "MN"=w485, "PW"=w486) -> ("错误常量"=w487:errorcluster, "通讯包字符串"=w483:string)  [unwired: 10 in]
                        n452 = call "通信状态入队列.vi"("错误输入（无错误）"=w487, "枚举"=enum16{"打开连接", "发送数据", "读取数据", "数据处理", "关闭连接"}."发送数据") -> ()  [unwired: 9 in, 1 out]
                        n453 = global write "全局1.vi" "发送报文显示"(w483) -> ()
                      }
                    }
                    n454 = global write "全局1.vi" "测量周期"(FALSE ("系统状态")) -> ()
                  }
                }
              }
              frame True {
              }
            }
          }
        }
      }
      frame "超标留样" {
        # "直接1分钟查询 一次,有变化就按上传,没变化就不上传"
        n455 = flat-sequence {
          frame #0 {
            # "时间"
            n456 = global write "全局 小时数据发送次数.vi" "小时数据发送次数"(0 ("小时数据发送次数")) -> ()
            n457 = global write "全局 数据数组大小.vi" "数据数组大小"(1 ("数据数组大小")) -> ()
            n458 = global write "全局1.vi" "枚举"(enum16{"返回请求应答", "上传数据", "返回执行结果"}."上传数据" ("枚举")) -> ()
          }
          frame #1 {
            # "判定是否存表"
            n459 = global read "全局 数据发送重叠.vi" "掉线指示灯"() -> (w492:bool)
            n460 = case shown="假" w492 {
              frame False {
                n461 = global read "全局1.vi" "超标留样"() -> (w493:bool)
                n462 = case shown="真" w493 {
                  frame False {
                  }
                  frame True {
                    n463 = global read "全局 小时数据发送次数.vi" "小时数据发送次数"() -> (w501:i32)
                    n464 = global write "全局1.vi" "超标留样"(FALSE ("系统状态")) -> ()
                    n465 = Get Date/Time In Seconds() -> (seconds since 1Jan1904=w505:timestamp)
                    n466 = Increment(x=w501) -> (x+1=w500:i32)
                    n467 = Format Date/Time String(time format string (%c)="%Y%m%d%H%M%S%3u" ("时间格式字符串(%c)"), seconds (now)=w505) -> (date/time string=w504:string)  [unwired: 1 in]
                    n468 = global write "全局 小时数据发送次数.vi" "小时数据发送次数"(w500) -> ()
                    n469 = Search and Replace String(input string=w504, search string="." ("搜索字符串")) -> (result string=w502:string)  [unwired: 6 in, 3 out]
                    n470 = global read "断电保存全局.vi" "MN"() -> (w496:string)
                    n471 = global read "断电保存全局.vi" "PW"() -> (w495:string)
                    n472 = call "数据编码.vi"("table输入"="超标留样" ("新元素/子数组"), "QN"=w502, "MN"=w496, "PW"=w495) -> ("错误常量"=w497:errorcluster, "通讯包字符串"=w499:string)  [unwired: 10 in]
                    n473 = global write "全局1.vi" "发送报文显示"(w499) -> ()
                    n474 = call "通信状态入队列.vi"("错误输入（无错误）"=w497, "枚举"=enum16{"打开连接", "发送数据", "读取数据", "数据处理", "关闭连接"}."发送数据") -> ()  [unwired: 9 in, 1 out]
                  }
                }
              }
              frame True {
              }
            }
          }
        }
      }
      frame "报警信息" {
        # "间隔时间上传"
        # "直接1分钟查询 一次,有数据就按数据上传,没数据为空的不传,在数据发送那边有做处理"
        n475 = flat-sequence {
          frame #0 {
            # "分钟时间间隔"
            n476 = call "日志信息主动发送(子VI).vi"() -> ()  [unwired: 12 in]
            n477 = global write "全局 小时数据发送次数.vi" "小时数据发送次数"(0 ("小时数据发送次数")) -> ()
            n478 = global write "全局1.vi" "枚举"(enum16{"返回请求应答", "上传数据", "返回执行结果"}."上传数据" ("枚举")) -> ()
          }
          frame #1 {
            n479 = call "获取报警信息 (子VI).vi"() -> ()  [unwired: 12 in]
          }
          frame #2 {
            n480 = call "数据处理整合 (子VI).vi"("枚举"=enum16{"实时数据排序", "小时数据排序"}."实时数据排序") -> ("已排序的数组"=w519:string[])  [unwired: 10 in]
            n481 = Array Size(array=w519) -> (size(s)=w518:i32)
            n482 = global write "全局 数据数组大小.vi" "数据数组大小"(w518) -> ()
          }
          frame #3 {
            n483 = global read "全局 数据发送重叠.vi" "掉线指示灯"() -> (w521:bool)
            n484 = Not(x=w521) -> (.not. x?=w520:bool)
            n485 = case shown="真" w520 {
              frame False {
              }
              frame True {
                n486 = global read "全局 时间2.vi" "报警信息索引"() -> (w525:T15)
                n487 = Cluster To Array(cluster=w525) -> (array=w524:string[])
                n488 = for {
                  tunnel: [w527] -> w522 mode=indexing
                  tunnel: w524 -> [w526] mode=indexing
                  i -> [w529]
                  # "行数大于零"
                  n489 = case shown="12" w529 {
                    tunnel: [w533 w534 w535 w536 w537 w538 w539 w540 w541 w542 w543 w544 w545] -> w528
                    frame 0, Default {
                      n490 = global read "全局 所有参数.vi" "氨氮"() -> (w533:string[][])
                    }
                    frame 1 {
                      n491 = global read "全局 所有参数.vi" "总磷"() -> (w534:string[][])
                    }
                    frame 2 {
                      n492 = global read "全局 所有参数.vi" "总氮"() -> (w535:string[][])
                    }
                    frame 3 {
                      n493 = global read "全局 所有参数.vi" "CODMn"() -> (w536:string[][])
                    }
                    frame 4 {
                      n494 = global read "全局 所有参数.vi" "CODCr"() -> (w537:string[][])
                    }
                    frame 5 {
                      n495 = global read "全局 所有参数.vi" "DO"() -> (w538:string[][])
                    }
                    frame 6 {
                      n496 = global read "全局 所有参数.vi" "PH"() -> (w539:string[][])
                    }
                    frame 7 {
                      n497 = global read "全局 所有参数.vi" "电导率"() -> (w540:string[][])
                    }
                    frame 8 {
                      n498 = global read "全局 所有参数.vi" "水温"() -> (w541:string[][])
                    }
                    frame 9 {
                      n499 = global read "全局 所有参数.vi" "浊度"() -> (w542:string[][])
                    }
                    frame 10 {
                      n500 = global read "全局 所有参数.vi" "叶绿素"() -> (w543:string[][])
                    }
                    frame 11 {
                      n501 = global read "全局 所有参数.vi" "藻密度"() -> (w544:string[][])
                    }
                    frame 12 {
                      n502 = global read "全局 所有参数.vi" "氟化物"() -> (w545:string[][])
                    }
                  }
                  n503 = Array Size(array=w528) -> (size(s)=w531:i32[])
                  n504 = Index Array(array=w531) -> (element=w530:i32)  [unwired: 1 in]
                  n505 = Greater Than 0?(x=w530) -> (x > 0?=w532:bool)
                  n506 = case shown="真" w532 {
                    tunnel: w530 -> [_ _]
                    tunnel: w528 -> [_ w550]
                    tunnel: [w546 w547] -> w527
                    tunnel: w526 -> [w546 _]
                    frame False {
                    }
                    frame True {
                      # "最新时间戳加1分钟"
                      n507 = Array Size(array=w550) -> (size(s)=w552:i32[])
                      n508 = Index Array(array=w552) -> (element=w551:i32)  [unwired: 1 in]
                      n509 = Decrement(x=w551) -> (x-1=w549:i32)
                      n510 = Index Array(array=w550, index (row)=w549, index (col)=0 ("禁用的索引 (列)")) -> (element=w553:string)
                      n511 = call "日期时间字符串转换分钟数加一.vi"("data[0]"=w553) -> ("日期/时间字符串"=w547:string)  [unwired: 10 in]
                    }
                  }
                }
                n512 = Array To Cluster(array=w522) -> (cluster=w523:T16)
                n513 = global write "全局 时间2.vi" "报警信息索引"(w523) -> ()
              }
            }
          }
          frame #4 {
            # "判定是否存表"
            n514 = global read "全局 数据发送重叠.vi" "掉线指示灯"() -> (w554:bool)
            n515 = case shown="假" w554 {
              frame False {
                # "判定数据不为空才发"
                n516 = global read "全局 数据数组大小.vi" "数据数组大小"() -> (w555:i32)
                n517 = Greater Than 0?(x=w555) -> (x > 0?=w556:bool)
                n518 = case shown="真" w556 {
                  frame False {
                    n519 = global write "全局1.vi" "核查数据上传"(FALSE ("数据上传")) -> ()
                  }
                  frame True {
                    n520 = while {
                      stop <- w559 stop-if-true
                      n521 = Wait (ms)(milliseconds to wait=u32 1000 ("等待时间（毫秒）")) -> ()  [unwired: 1 out]
                      n522 = Get Date/Time In Seconds() -> (seconds since 1Jan1904=w571:timestamp)
                      n523 = Format Date/Time String(time format string (%c)="%Y%m%d%H%M%S%3u" ("时间格式字符串(%c)"), seconds (now)=w571) -> (date/time string=w570:string)  [unwired: 1 in]
                      n524 = global read "全局 数据数组大小.vi" "数据数组大小"() -> (w561:i32)
                      n525 = Search and Replace String(input string=w570, search string="." ("搜索字符串")) -> (result string=w568:string)  [unwired: 6 in, 3 out]
                      n526 = global read "断电保存全局.vi" "PW"() -> (w564:string)
                      n527 = global read "断电保存全局.vi" "MN"() -> (w565:string)
                      n528 = global read "全局 小时数据发送次数.vi" "小时数据发送次数"() -> (w562:i32)
                      n529 = call "数据编码.vi"("table输入"="报警信息" ("新元素/子数组"), "QN"=w568, "MN"=w565, "PW"=w564) -> ("错误常量"=w563:errorcluster, "通讯包字符串"=w567:string)  [unwired: 10 in]
                      n530 = Decrement(x=w561) -> (x-1=w560:i32)
                      n531 = global write "全局1.vi" "发送报文显示"(w567) -> ()
                      n532 = Greater Or Equal?(x=w562, y=w560) -> (x >= y?=w559:bool)
                      n533 = call "通信状态入队列.vi"("错误输入（无错误）"=w563, "枚举"=enum16{"打开连接", "发送数据", "读取数据", "数据处理", "关闭连接"}."发送数据") -> ()  [unwired: 9 in, 1 out]
                    }
                  }
                }
              }
              frame True {
              }
            }
          }
        }
        n534 = global read "断电保存全局.vi" "应用环境"() -> (w509:enum16{"STD", "GB212"})
        n535 = case shown="\"GB212\"" w509 {
          tunnel: ["3093报警信息" ("组合框") w512] -> w508
          frame "STD", Default {
          }
          frame "GB212" {
            n536 = global read "断电保存全局.vi" "仪器参数发送"() -> (w511:bool)
            n537 = case shown="假" w511 {
              tunnel: ["环境参数" ("组合框") "仪器参数" ("组合框")] -> w512
              frame False {
              }
              frame True {
              }
            }
          }
        }
      }
      frame "3093报警信息" {
        # "间隔时间上传"
        # "直接1分钟查询 一次,有数据就按数据上传,没数据为空的不传,在数据发送那边有做处理"
        n538 = flat-sequence {
          tunnel: [w581] -> w576
          tunnel: w576 -> [w585]
          frame #0 {
            n539 = global write "全局 小时数据发送次数.vi" "小时数据发送次数"(0 ("小时数据发送次数")) -> ()
            n540 = global write "全局1.vi" "枚举"(enum16{"返回请求应答", "上传数据", "返回执行结果"}."上传数据" ("枚举")) -> ()
          }
          frame #1 {
            n541 = call "数据表比对.vi"("table输入"="3093报警信息") -> ("待发送数据"=w581:string[][])  [unwired: 7 in, 3 out]
            n542 = global write "全局 所有参数.vi" "CODMn"(w581) -> ()
          }
          frame #2 {
            n543 = Array Size(array=w585) -> (size(s)=w584:i32[])
            n544 = Index Array(array=w584) -> (element=w583:i32)  [unwired: 1 in]
            n545 = global write "全局 数据数组大小.vi" "数据数组大小"(w583) -> ()
          }
          frame #3 {
            n546 = global read "全局 数据发送重叠.vi" "掉线指示灯"() -> (w587:bool)
            n547 = Not(x=w587) -> (.not. x?=w586:bool)
            n548 = case shown="真" w586 {
              frame False {
              }
              frame True {
                # "行数大于零"
                n549 = global read "全局 时间2.vi" "3093报警索引起始时间"() -> (w589:string)
                n550 = global read "全局 所有参数.vi" "CODMn"() -> (w590:string[][])
                n551 = Array Size(array=w590) -> (size(s)=w592:i32[])
                n552 = Index Array(array=w592) -> (element=w591:i32)  [unwired: 1 in]
                n553 = Greater Than 0?(x=w591) -> (x > 0?=w593:bool)
                n554 = case shown="真" w593 {
                  tunnel: w591 -> [_ _]
                  tunnel: w590 -> [_ w599]
                  tunnel: [w594 w595] -> w588
                  tunnel: w589 -> [w594 _]
                  frame False {
                  }
                  frame True {
                    # "最新时间戳加1分钟"
                    n555 = Array Size(array=w599) -> (size(s)=w601:i32[])
                    n556 = Index Array(array=w601) -> (element=w600:i32)  [unwired: 1 in]
                    n557 = Decrement(x=w600) -> (x-1=w598:i32)
                    n558 = Index Array(array=w599, index (row)=w598, index (col)=0 ("禁用的索引 (列)")) -> (element=w596:string)
                    n559 = call "日期时间字符串转换秒数加一.vi"("data[0]"=w596) -> ("日期/时间字符串"=w595:string)  [unwired: 10 in]
                  }
                }
                n560 = global write "全局 时间2.vi" "3093报警索引起始时间"(w588) -> ()
              }
            }
          }
          frame #4 {
            # "判定是否存表"
            n561 = global read "全局 数据发送重叠.vi" "掉线指示灯"() -> (w602:bool)
            n562 = case shown="假" w602 {
              frame False {
                n563 = global read "全局 数据数组大小.vi" "数据数组大小"() -> (w603:i32)
                n564 = Greater Than 0?(x=w603) -> (x > 0?=w604:bool)
                n565 = case shown="真" w604 {
                  frame False {
                  }
                  frame True {
                    n566 = while {
                      stop <- w606 stop-if-true
                      n567 = global read "全局 数据数组大小.vi" "数据数组大小"() -> (w608:i32)
                      n568 = Wait (ms)(milliseconds to wait=u32 1000 ("等待时间（毫秒）")) -> ()  [unwired: 1 out]
                      n569 = global read "全局 小时数据发送次数.vi" "小时数据发送次数"() -> (w607:i32)
                      n570 = Decrement(x=w608) -> (x-1=w609:i32)
                      n571 = Greater Or Equal?(x=w607, y=w609) -> (x >= y?=w606:bool)
                      n572 = Get Date/Time In Seconds() -> (seconds since 1Jan1904=w618:timestamp)
                      n573 = Format Date/Time String(time format string (%c)="%Y%m%d%H%M%S%3u" ("时间格式字符串(%c)"), seconds (now)=w618) -> (date/time string=w617:string)  [unwired: 1 in]
                      n574 = Search and Replace String(input string=w617, search string="." ("搜索字符串")) -> (result string=w615:string)  [unwired: 6 in, 3 out]
                      n575 = global read "断电保存全局.vi" "MN"() -> (w612:string)
                      n576 = global read "断电保存全局.vi" "PW"() -> (w611:string)
                      n577 = call "数据编码.vi"("table输入"="3093报警信息" ("新元素/子数组"), "QN"=w615, "MN"=w612, "PW"=w611) -> ("错误常量"=w610:errorcluster, "通讯包字符串"=w614:string)  [unwired: 10 in]
                      n578 = call "通信状态入队列.vi"("错误输入（无错误）"=w610, "枚举"=enum16{"打开连接", "发送数据", "读取数据", "数据处理", "关闭连接"}."发送数据") -> ()  [unwired: 9 in, 1 out]
                      n579 = global write "全局1.vi" "发送报文显示"(w614) -> ()
                    }
                  }
                }
              }
              frame True {
              }
            }
          }
        }
        n580 = global read "断电保存全局.vi" "仪器参数发送"() -> (w575:bool)
        n581 = case shown="假" w575 {
          tunnel: ["环境参数" ("组合框") "仪器参数" ("组合框")] -> w574
          frame False {
          }
          frame True {
          }
        }
      }
      frame "仪器参数" {
        n582 = flat-sequence {
          frame #0 {
            n583 = global write "全局 小时数据发送次数.vi" "小时数据发送次数"(0 ("小时数据发送次数")) -> ()
            n584 = global write "全局1.vi" "枚举"(enum16{"返回请求应答", "上传数据", "返回执行结果"}."上传数据" ("枚举")) -> ()
          }
          frame #1 {
            n585 = call "获取操作日志 (子VI).vi"("table输入"="仪器参数") -> ()  [unwired: 11 in]
          }
          frame #2 {
            n586 = global read "全局 数据发送重叠.vi" "掉线指示灯"() -> (w626:bool)
            n587 = Not(x=w626) -> (.not. x?=w625:bool)
            n588 = case shown="真" w625 {
              frame False {
              }
              frame True {
                n589 = global read "全局 时间2.vi" "仪器参数索引"() -> (w630:T17)
                n590 = Cluster To Array(cluster=w630) -> (array=w629:string[])
                n591 = for {
                  tunnel: [w634] -> w627 mode=indexing
                  tunnel: w629 -> [w633] mode=indexing
                  i -> [w632]
                  # "行数大于零"
                  n592 = case shown="13" w632 {
                    tunnel: [w638 w639 w640 w641 w642 w643 w644 w645 w646 w647 w648 w649 w650 w651] -> w631
                    frame 0, Default {
                      n593 = global read "全局 所有参数.vi" "氨氮"() -> (w638:string[][])
                    }
                    frame 1 {
                      n594 = global read "全局 所有参数.vi" "总磷"() -> (w639:string[][])
                    }
                    frame 2 {
                      n595 = global read "全局 所有参数.vi" "总氮"() -> (w640:string[][])
                    }
                    frame 3 {
                      n596 = global read "全局 所有参数.vi" "CODMn"() -> (w641:string[][])
                    }
                    frame 4 {
                      n597 = global read "全局 所有参数.vi" "CODCr"() -> (w642:string[][])
                    }
                    frame 5 {
                      n598 = global read "全局 所有参数.vi" "DO"() -> (w643:string[][])
                    }
                    frame 6 {
                      n599 = global read "全局 所有参数.vi" "PH"() -> (w644:string[][])
                    }
                    frame 7 {
                      n600 = global read "全局 所有参数.vi" "电导率"() -> (w645:string[][])
                    }
                    frame 8 {
                      n601 = global read "全局 所有参数.vi" "水温"() -> (w646:string[][])
                    }
                    frame 9 {
                      n602 = global read "全局 所有参数.vi" "浊度"() -> (w647:string[][])
                    }
                    frame 10 {
                      n603 = global read "全局 所有参数.vi" "叶绿素"() -> (w648:string[][])
                    }
                    frame 11 {
                      n604 = global read "全局 所有参数.vi" "藻密度"() -> (w649:string[][])
                    }
                    frame 12 {
                      n605 = global read "全局 所有参数.vi" "ORP"() -> (w650:string[][])
                    }
                    frame 13 {
                      n606 = global read "全局 所有参数.vi" "氟化物"() -> (w651:string[][])
                    }
                  }
                  n607 = Array Size(array=w631) -> (size(s)=w636:i32[])
                  n608 = Index Array(array=w636) -> (element=w635:i32)  [unwired: 1 in]
                  n609 = Greater Than 0?(x=w635) -> (x > 0?=w637:bool)
                  n610 = case shown="真" w637 {
                    tunnel: w635 -> [_ _]
                    tunnel: w631 -> [_ w657]
                    tunnel: [w652 w654] -> w634
                    tunnel: w633 -> [w652 _]
                    frame False {
                    }
                    frame True {
                      # "最新时间戳加1秒"
                      n611 = Array Size(array=w657) -> (size(s)=w659:i32[])
                      n612 = Index Array(array=w659) -> (element=w658:i32)  [unwired: 1 in]
                      n613 = Decrement(x=w658) -> (x-1=w656:i32)
                      n614 = Index Array(array=w657, index (row)=w656, index (col)=0 ("禁用的索引 (列)")) -> (element=w660:string)
                      n615 = call "日期时间字符串转换分钟数加一.vi"("枚举"=enum16{"分钟数加一", "秒数加一", "小时数加一"}."秒数加一", "data[0]"=w660) -> ("日期/时间字符串"=w654:string)  [unwired: 9 in]
                    }
                  }
                }
                n616 = Array To Cluster(array=w627) -> (cluster=w628:T18)
                n617 = global write "全局 时间2.vi" "仪器参数索引"(w628) -> ()
              }
            }
          }
          frame #3 {
            n618 = global read "全局 数据发送重叠.vi" "掉线指示灯"() -> (w662:bool)
            n619 = Not(x=w662) -> (.not. x?=w661:bool)
            n620 = case shown="真" w661 {
              frame False {
              }
              frame True {
                n621 = call "3020仪器参数发送.vi"() -> ()  [unwired: 12 in]
              }
            }
          }
        }
      }
      frame "环境参数", Default {
        n622 = call "核查数据断电保存 (子VI).vi"() -> ()  [unwired: 12 in]
      }
    }
  }
  "错误输出" <- w2
